vi "LaserPanel.vi"() -> ()   [LabVIEW 2014]
uses:
  <vilib>/event_ctls.llb/eventvkey.ctl
  <vilib>/Instr/_visa.llb/VISA Configure Serial Port (Instr).vi
  wlmData.dll
panel:
  out "Oscilloscope Error":errorcluster
  in  "RF Low":bool=TRUE
  out "Numeric":dbl
  out "Saes Error":errorcluster
  out "Ion\nPump":string="0 nA"
  out "Trap RF error":errorcluster
  out "Horn Error":errorcluster
  out "Cureent error":errorcluster
  out "Oven error":errorcluster
  out "aruduino error":errorcluster
  out "PMT 2":dbl=70.0 format="%.2f"
  in  "DeviceTab":T1(tab)
  in  "Brightness":dbl=30.0
  out "ERROR":string
  in  "Show WLM APP":bool=TRUE
  in  "stop 2":bool
  in  "Expo.[ms]":i32[](array[numeric])
  out "Pattern":i16[][](graph)
  out "Pattern2":i16[][](graph)
  in  "Auto":bool
  in  "Use":bool=TRUE
  in  "stop 3":bool
  out "PID Warning":bool
  out "Act Wavelength (nm)":string
  in  "PID gains":T2={"Pg (Kc)"=1000.0, "It (Ti, min)"=0.0, "Dt (Td, min)"=0.0} {"Dt (Td, min)" format="%.3f"; "It (Ti, min)" format="%.3f"; "Pg (Kc)" format="%.3f"}
  out "Warning":bool
  in  "Set Voltage (V)":dbl=70.0 min=50.0 max=90.0 format="%.3f"
  in  "Set Current  (mA)":dbl=70.0 format="%.3f"
  in  "Set Temperature":dbl=70.0 format="%.3f"
  out "Act Voltage (V)":dbl=70.0 format="%.3f"
  in  "Laser":i16(ring) items=["370", "399", "729", "935"]
  in  "Lock":bool
  in  "Set Wavelength (nm)":dbl=70.0 format="%.6f"
  out "Act Current (mA)":dbl=70.0 format="%.1f"
  out "Max Current (mA)":dbl=70.0 format="%.3f"
  out "Act Temperature":dbl=70.0 format="%.3f"
  in  "RF OFF":bool=TRUE
  in  "Oven+399/SPACE":bool
  in  "Ion refind":bool
  in  "Ion Capture":bool
  out "output 1":dbl
  in  "Ch2 Scale":dbl(ring)=0.5 items=["10V"=10.0, "5V"=5.0, "2V"=2.0, "1V"=1.0, "500mV"=0.5, "200mV"=0.2, "100mV"=0.1, "50mV"=0.05, "20mV"=0.02, "10mV"=0.01, "5mV"=0.005, "2mV"=0.002, "1mV"=0.001]
  out "Numeric 2":dbl
  out "Ch2 pk-pk(V)":dbl format="%.3f"
  out "Ch1 pk-pk(V)":dbl format="%.3f"
  out "ERROR2":string caption="ERROR"
  out "trap default":dbl
  in  "VISA Input":string
  out "VISA Output":string
  in  "Amplitude (dBm)":dbl format="%.1f"
  in  "RFon/off":bool caption="ON"
  in  "Amplitude2(dBm)":dbl format="%.1f"
  in  "Frequency (MHz)":dbl format="%.4f"
  in  "Device":i16(ring) items=["Trap", "Horn/Raman"]
  out "ERROR3":string caption="ERROR"
  in  "Track":i16(ring) items=["Indenpent", "Series", "Parallel"]
  out "Temperature":dbl format="%.2f"
  in  "Channel":i16(ring) items=["Oven", "Current1", "Current2", "Current3", "Current4"]
  in  "Con/off":bool caption="ON"
  out "T":dbl(slide) scale=0.0..100.0
  out "CV":bool
  out "CC":bool
  in  "Set Voltage (V)":dbl=1.5 format="%.3f"
  in  "Set Current (A)":dbl=1.3 format="%.3f"
  out "Act Voltage (V)":dbl format="%.3f"
  out "Act Current (A)":dbl format="%.3f"
  out "PMT":dbl=70.0 format="%.2f"
  in  "CCD/F7":bool=TRUE
  in  "935/F6":bool=TRUE
  in  "399":bool=TRUE
  in  "370/F5":bool=TRUE
  in  "Show2":bool=TRUE
  in  "Show4":bool=TRUE
  in  "Show1":bool=TRUE
  in  "Show3":bool=TRUE
  out "Booleanno":bool
  out "Boolean 2":bool
  out "Boolean":bool
  in  "Warning 3":bool
  in  "Warning 2":bool
  in  "Warning 1":bool
  in  "Warning 0":bool
  out "Set Volt Array 0":dbl[](array[numeric])
  out "935":string
  out "729":string
  out "399":string
  out "370":string
  out "Act Wavelength number (nm)":dbl=70.0 format="%.6f"
  out "Set wave Array":dbl[](array[numeric])
  out "Lock Array":bool[](array[boolean])
  in  "stop":bool
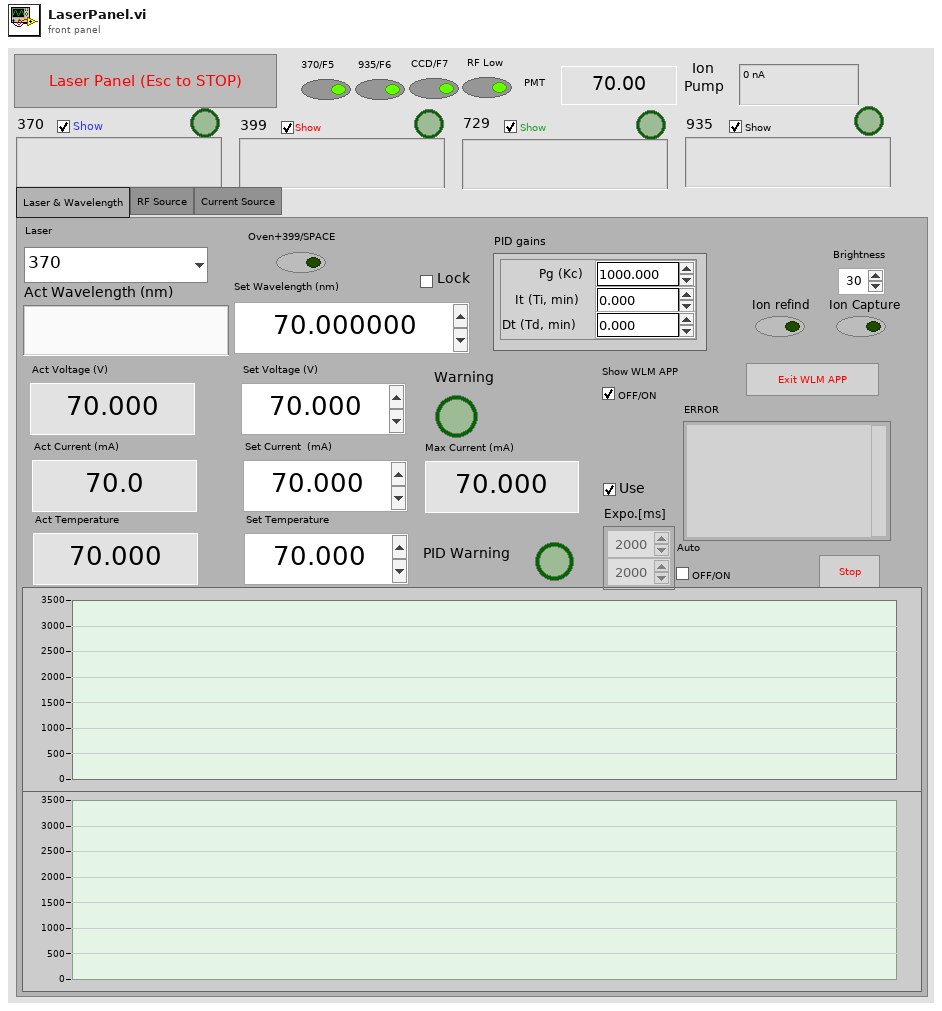
[diagram p1: front panel]
types:
  T1 = enum32{"Laser & Wavelength", "RF Source", "Current Source"}
  T2 = cluster{"Pg (Kc)":dbl, "It (Ti, min)":dbl, "Dt (Td, min)":dbl}
  T3 = typedef "eventvkey.ctl" = enum16{"ASCII", "Enter", "Return", "Shift", "Ctrl", "Alt", "Cmd", "Opt", "Caps", "NumLock", "Clear", "Break", "Up", "Down", "Left", "Right", "Insert", "Delete", "Home", "End", "PageUp", "PageDown", "Escape", "Help", "Pause", "ScrollLock", "F1", "F2", "F3", "F4", "F5", "F6", "F7", "F8", "F9", "F10", "F11", "F12", "F13", "F14", "F15", "F16", "F17", "F18", "F19", "F20", "F21", "F22", "F23", "F24", "Play", "VolumeUp", "VolumeDown", "Mute", "Two Byte Char"}
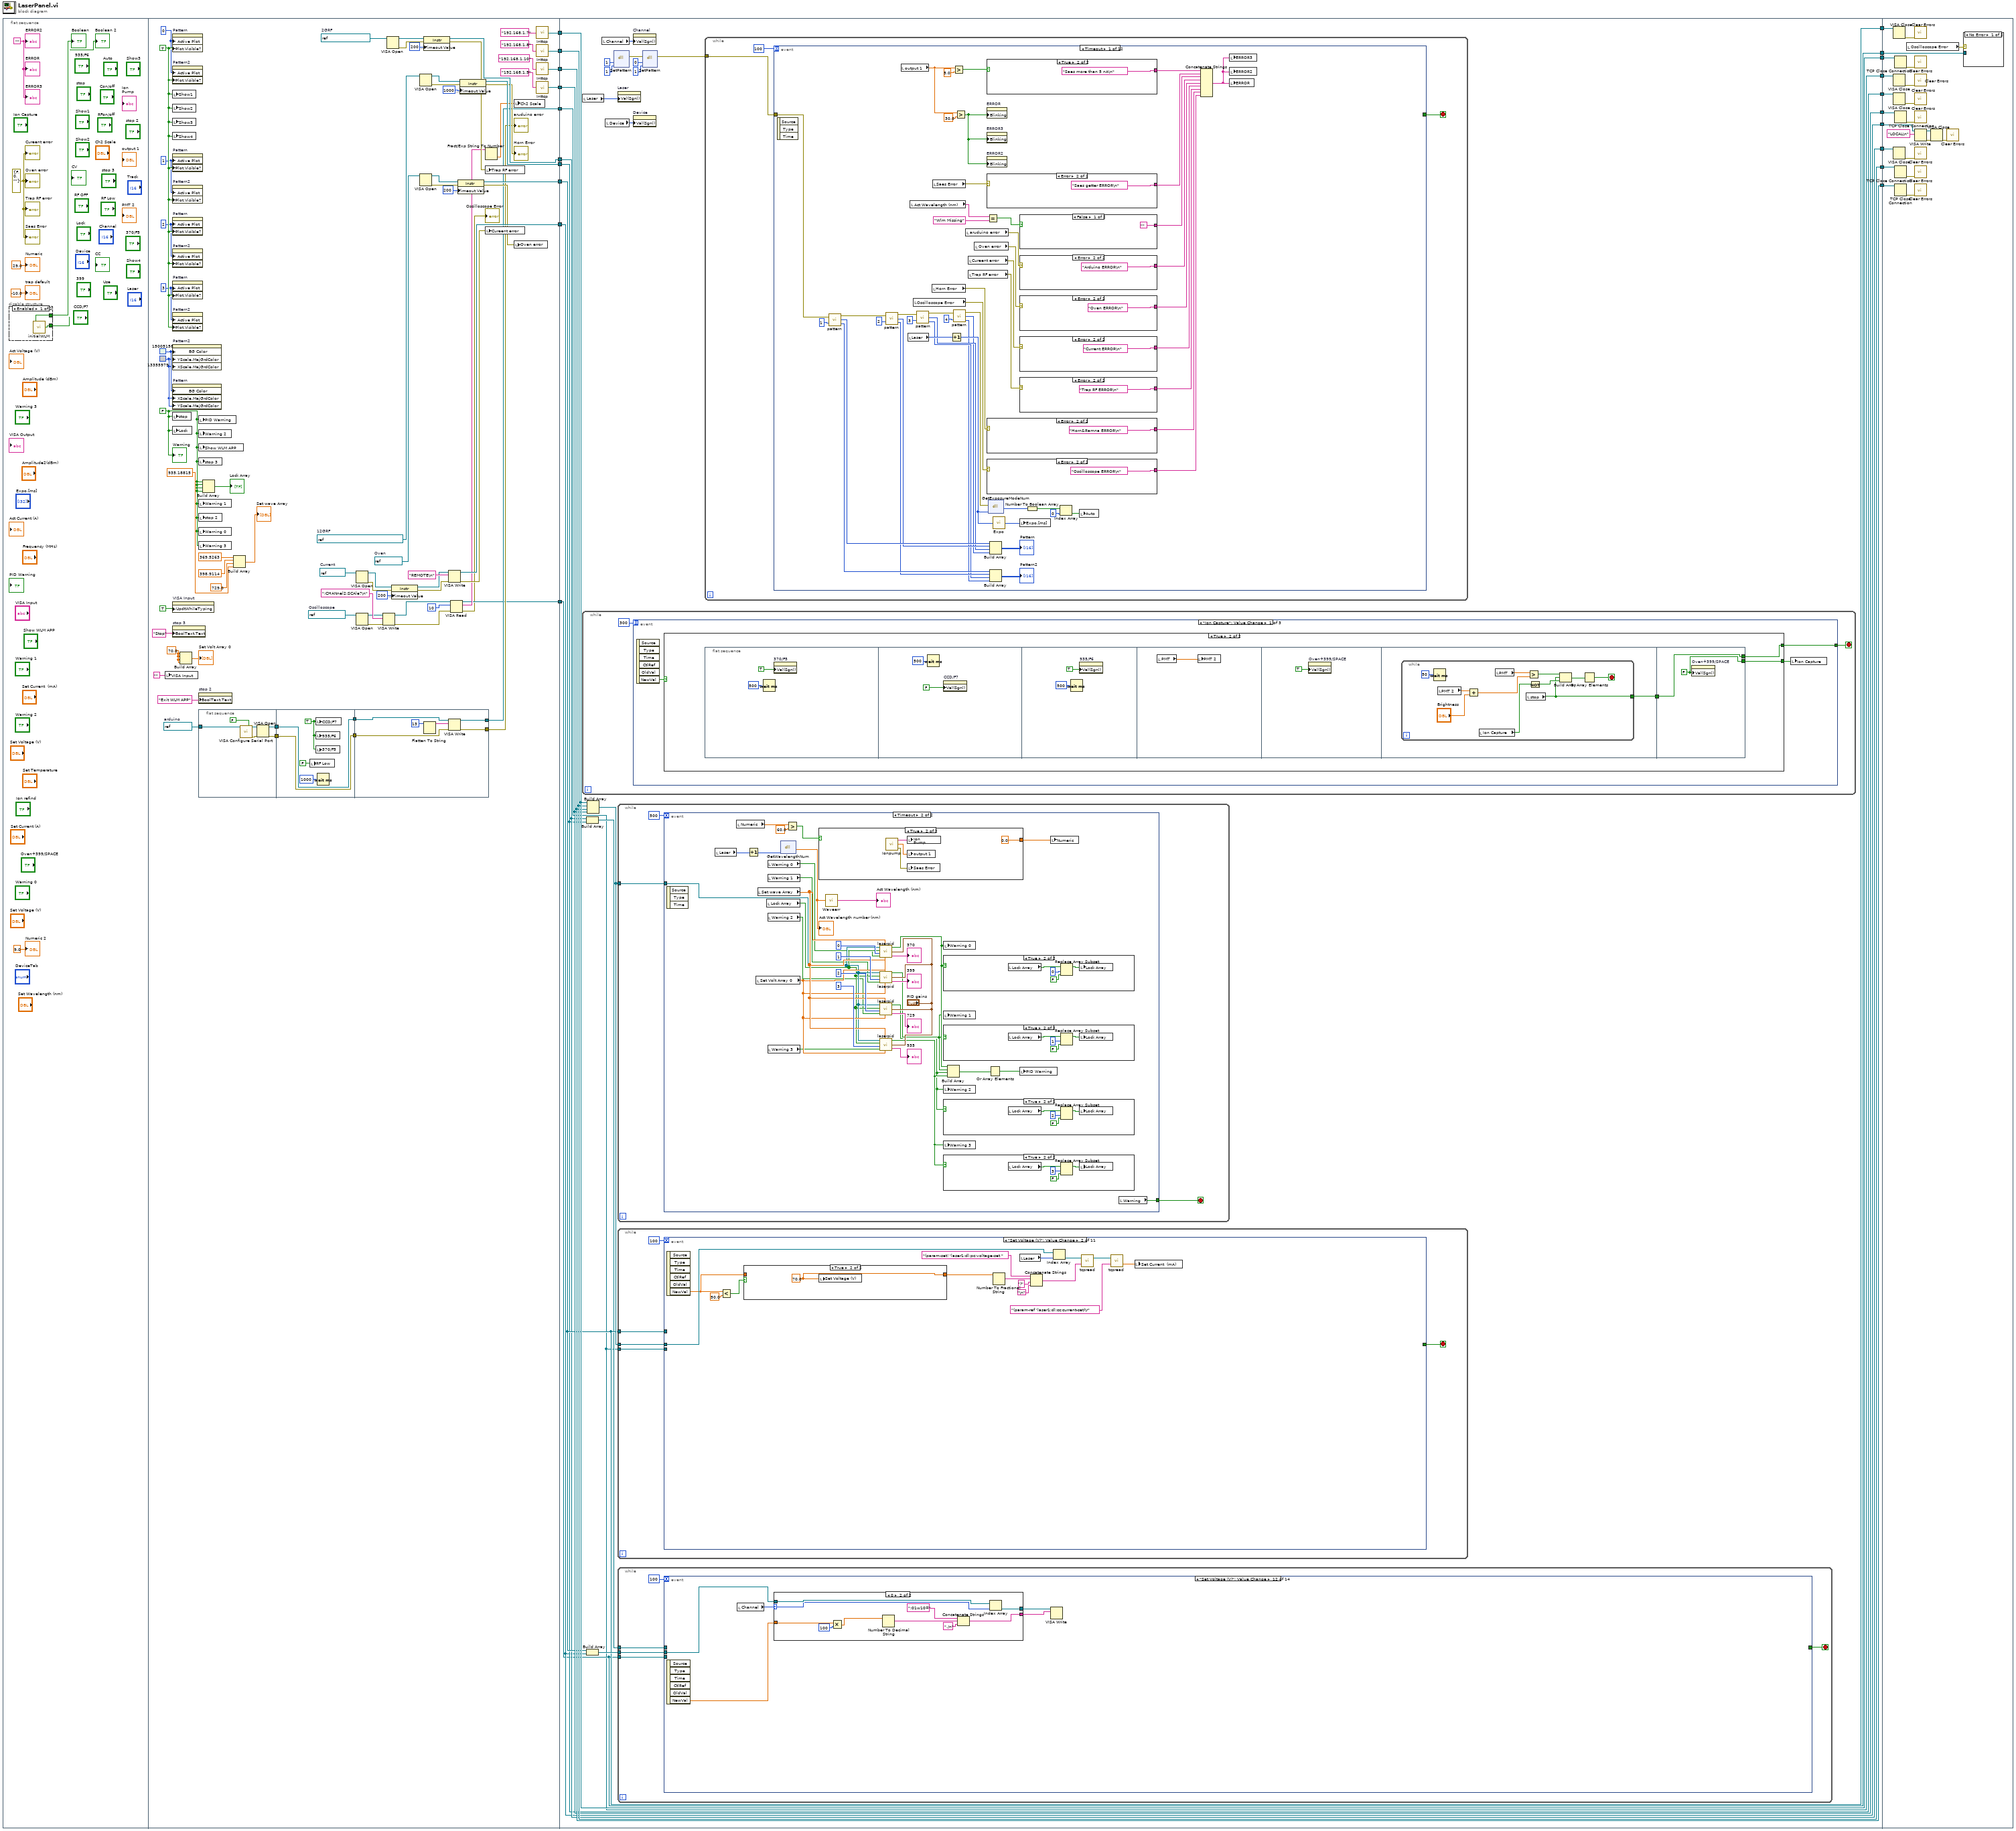
[diagram p0: block diagram]
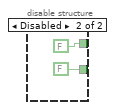
[diagram p2: hidden frame]
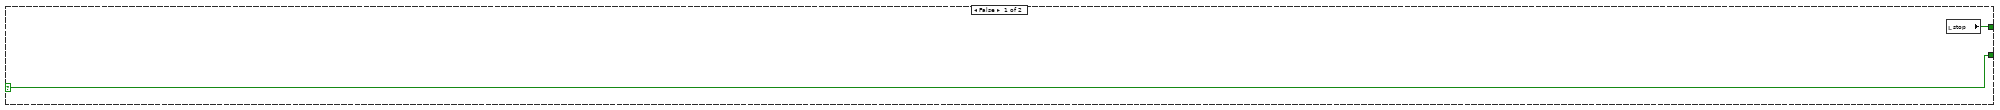
[diagram p3: hidden frame]
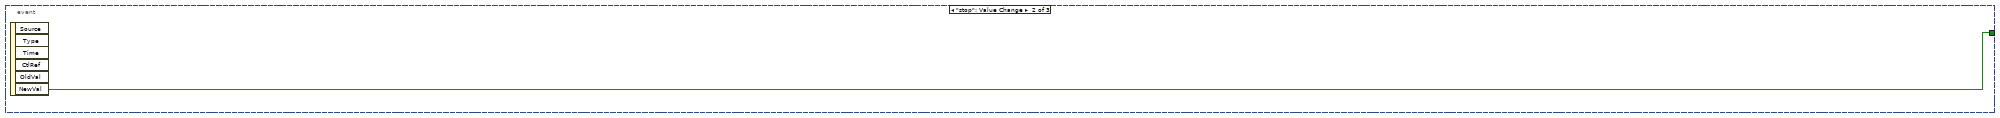
[diagram p4: hidden frame]
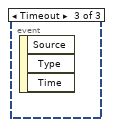
[diagram p5: hidden frame]
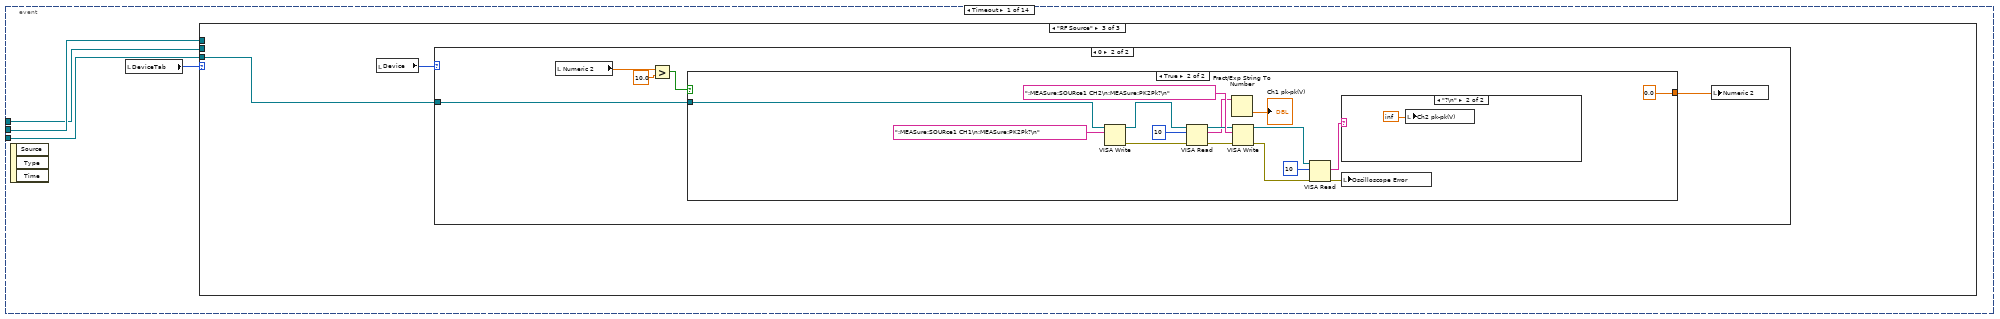
[diagram p6: hidden frame]
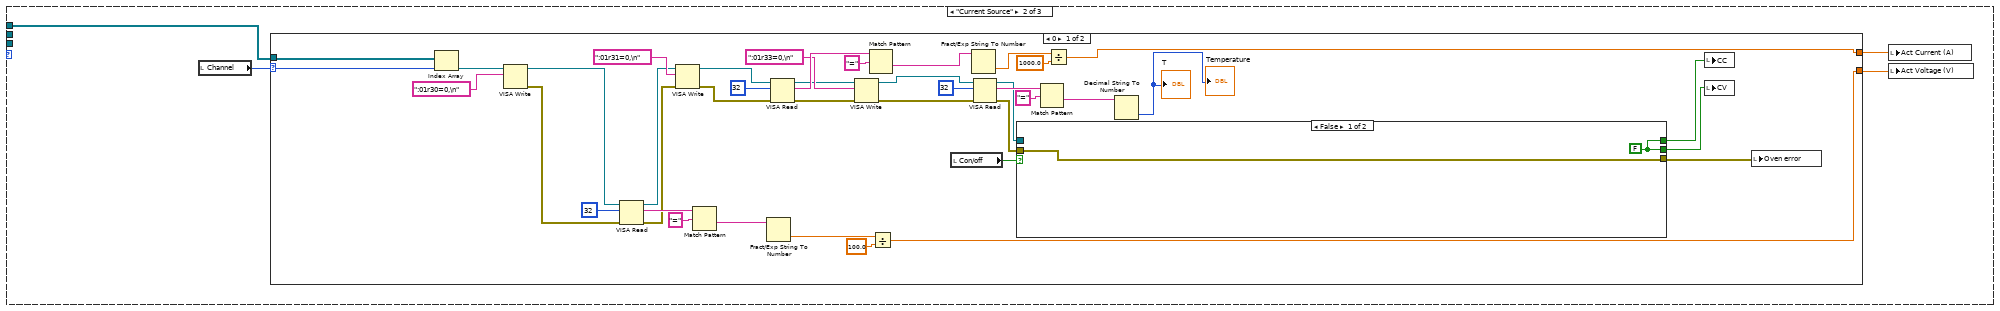
[diagram p8: hidden frame]
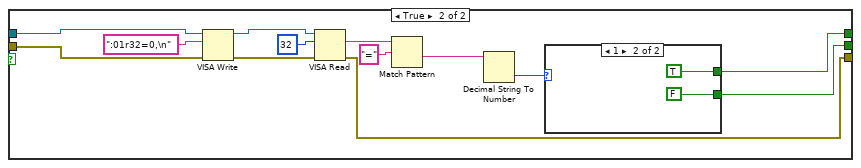
[diagram p9: hidden frame]
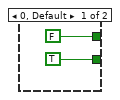
[diagram p10: hidden frame]
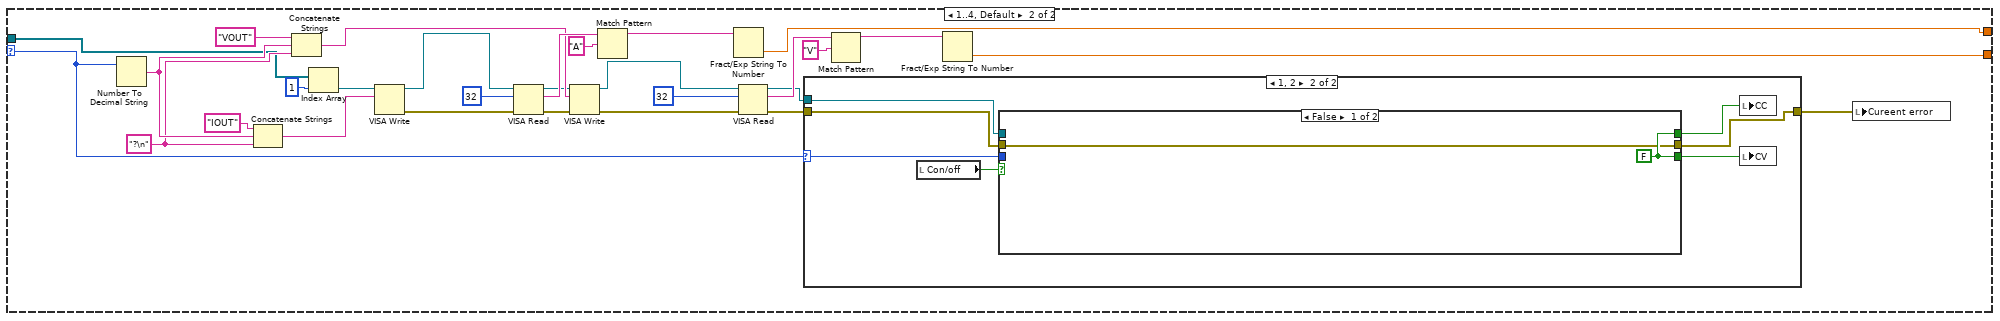
[diagram p11: hidden frame]
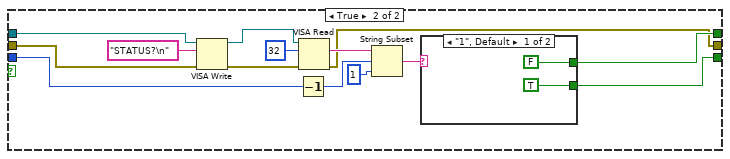
[diagram p13: hidden frame]
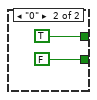
[diagram p14: hidden frame]
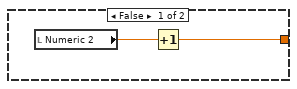
[diagram p16: hidden frame]
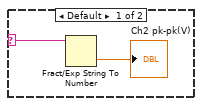
[diagram p17: hidden frame]
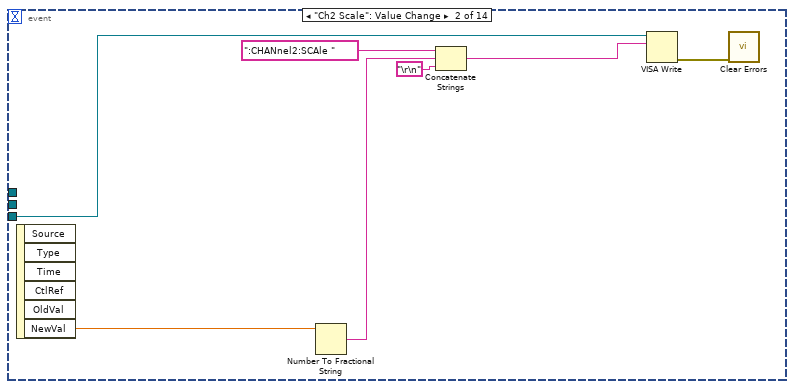
[diagram p18: hidden frame]
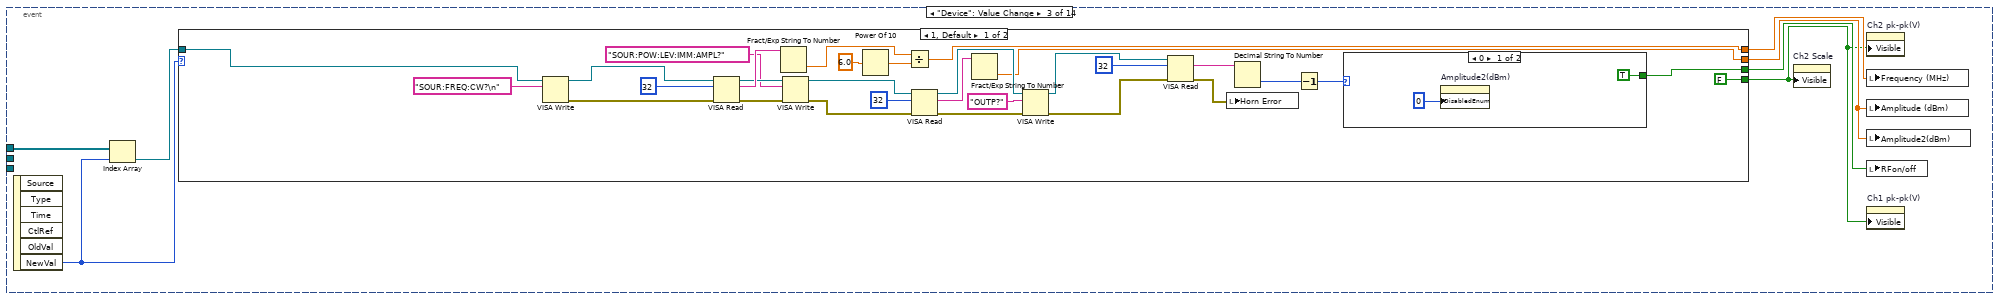
[diagram p19: hidden frame]
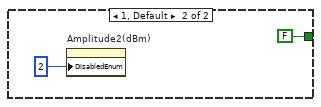
[diagram p20: hidden frame]
diagram:
  n1 = flat-sequence {
    tunnel: [w102] -> w20
    tunnel: [w101] -> w19
    tunnel: [w100] -> w18
    tunnel: [w99] -> w17
    tunnel: [w45] -> w12
    tunnel: [w57] -> w11
    tunnel: [w61] -> w10
    tunnel: [w69] -> w6
    tunnel: [w60] -> w4
    tunnel: [w37] -> w2
    tunnel: w20 -> [w142]
    tunnel: w19 -> [w141]
    tunnel: w18 -> [w140]
    tunnel: w17 -> [w139]
    tunnel: [w142] -> w16
    tunnel: [w141] -> w15
    tunnel: [w140] -> w14
    tunnel: [w139] -> w13
    tunnel: w12 -> [w122]
    tunnel: w11 -> [w130]
    tunnel: w10 -> [w129]
    tunnel: [w122] -> w9
    tunnel: [w130] -> w8
    tunnel: [w129] -> w7
    tunnel: w6 -> [w125]
    tunnel: [w125] -> w5
    tunnel: w4 -> [w124]
    tunnel: [w124] -> w3
    tunnel: w2 -> [w123]
    tunnel: [w123] -> w1
    tunnel: w16 -> [w1110]
    tunnel: w15 -> [w1109]
    tunnel: w14 -> [w1108]
    tunnel: w13 -> [w1107]
    tunnel: w9 -> [w1106]
    tunnel: w8 -> [w1105]
    tunnel: w7 -> [w1104]
    tunnel: w5 -> [w1103]
    tunnel: w3 -> [w1101]
    tunnel: w1 -> [w1099]
    frame #0 {
      w22 = ""
      w24 = errorcluster {"status"=FALSE, "code"=0, "source"=""} ("aruduino error 4")
      n2 = disable-structure shown="Enabled" {
        disable-tunnel: [w29 FALSE] -> w27
        disable-tunnel: [w28 FALSE] -> w26
        frame Enabled {
          n3 = call "initialWLM.vi"() -> ("Boolean 2"=w28:bool, "Boolean"=w29:bool)
        }
        frame Disabled {
        }
      }
      "Boolean" <- w27
      "Boolean 2" <- w26
      "trap default" <- -10.0
      "ERROR" <- w22
      "Trap RF error" <- w24
      "Cureent error" <- w24
      "Oven error" <- w24
      "ERROR2" <- w22
      "ERROR3" <- w22
      "Saes Error" <- w24
      "Numeric" <- 29.0
      "Numeric 2" <- 9.0
    }
    frame #1 {
      w52 = refnum<visa-resource-name> "GDS-1104B"  # Oscilloscope
      w68 = refnum<visa-resource-name> "COM7"  # Current
      w72 = refnum<visa-resource-name> "TCPIP0::192.168.1.11::inst0::INSTR"  # 12GRF
      w77 = refnum<visa-resource-name> "GPIB0::28::INSTR"  # 2GRF
      w78 = refnum<visa-resource-name> "COM16"  # Oven
      w79 = refnum<visa-resource-name> "COM21"  # arduino
      w84 = TRUE
      w81 = 2
      w80 = 3
      w82 = 1
      w83 = 0
      w87 = u32 13355979 ("Color Box")
      w88 = u32 15005158
      w91 = 70.0
      w48 = FALSE
      n4 = local write "VISA Input"("") -> ()
      n5 = property on="Pattern" class="WFGraph (strict)"("Active Plot"=w83, "Plot.Visible?"=w84) -> ()  [unwired: 2 in, 2 out]
      n6 = property on="Pattern2" class="WFGraph (strict)"("Active Plot"=w83, "Plot.Visible?"=w84) -> ()  [unwired: 2 in, 2 out]
      n7 = local write "Show1"(w84) -> ()
      n8 = local write "Show2"(w84) -> ()
      n9 = local write "Show3"(w84) -> ()
      n10 = local write "Show4"(w84) -> ()
      n11 = property on="Pattern" class="WFGraph (strict)"("Active Plot"=w82, "Plot.Visible?"=w84) -> ()  [unwired: 2 in, 2 out]
      n12 = property on="Pattern2" class="WFGraph (strict)"("Active Plot"=w82, "Plot.Visible?"=w84) -> ()  [unwired: 2 in, 2 out]
      n13 = property on="Pattern" class="WFGraph (strict)"("Active Plot"=w81, "Plot.Visible?"=w84) -> ()  [unwired: 2 in, 2 out]
      n14 = property on="Pattern2" class="WFGraph (strict)"("Active Plot"=w81, "Plot.Visible?"=w84) -> ()  [unwired: 2 in, 2 out]
      n15 = property on="Pattern" class="WFGraph (strict)"("Active Plot"=w80, "Plot.Visible?"=w84) -> ()  [unwired: 2 in, 2 out]
      n16 = property on="Pattern2" class="WFGraph (strict)"("Active Plot"=w80, "Plot.Visible?"=w84) -> ()  [unwired: 2 in, 2 out]
      n17 = property on="Pattern2" class="WFGraph (strict)"("BG Color"=w88, "YScale.MajGrdColor"=w87, "XScale.MajGrdColor"=w87) -> ()  [unwired: 2 in, 2 out]
      n18 = property on="Pattern" class="WFGraph (strict)"("BG Color"=w88, "XScale.MajGrdColor"=w87, "YScale.MajGrdColor"=w87) -> ()  [unwired: 2 in, 2 out]
      n19 = local write "stop"(w48) -> ()
      n20 = local write "Lock"(w48) -> ()
      n21 = property on="VISA Input" class="Str"("UpdtWhileTyping"=TRUE) -> ()  [unwired: 2 in, 2 out]
      n22 = property on="stop 3" class="Bool (strict)"("BoolText.Text"="Stop") -> ()  [unwired: 2 in, 2 out]
      n23 = Build Array(w91, w91, w91, w91) -> (→"Set Volt Array 0":dbl[])
      n24 = local write "PID Warning"(w48) -> ()
      n25 = local write "Warning 2"(w48) -> ()
      n26 = local write "Show WLM APP"(w48) -> ()
      n27 = local write "stop 3"(w48) -> ()
      n28 = local write "Warning 1"(w48) -> ()
      n29 = local write "stop 2"(w48) -> ()
      n30 = local write "Warning 0"(w48) -> ()
      n31 = local write "Warning 3"(w48) -> ()
      n32 = property on="stop 2" class="Bool (strict)"("BoolText.Text"="Exit WLM APP") -> ()  [unwired: 2 in, 2 out]
      n33 = flat-sequence {
        tunnel: w79 -> [w110]
        tunnel: [w106] -> w46
        tunnel: [w105] -> w43
        tunnel: [w115] -> w47
        tunnel: w46 -> [w115]
        tunnel: [w111] -> w44
        tunnel: w43 -> [w111]
        tunnel: w47 -> [w119]
        tunnel: [w118] -> w45
        tunnel: w44 -> [w117]
        tunnel: [w116] -> w42
        frame #0 {
          n34 = call-poly "VISA Configure Serial Port"("VISA resource name"=w110, "Enable Termination\nChar (T)"=FALSE ("Enable Termination\nChar (T)")) -> ("VISA resource name out"=w108:refnum<visa-resource-name>, "error out"=w107:errorcluster)  [unwired: 12 in]
          n35 = VISA Open(error in (no error)=w107, VISA resource name=w108) -> (VISA resource name=w106:refnum<visa-resource-name>, error out=w105:errorcluster)  [unwired: 3 in]
        }
        frame #1 {
          w113 = TRUE
          n36 = local write "RF Low"(FALSE) -> ()
          n37 = local write "CCD/F7"(w113) -> ()
          n38 = local write "935/F6"(w113) -> ()
          n39 = local write "370/F5"(w113) -> ()
          n40 = Wait (ms)(milliseconds to wait=u32 1000) -> ()  [unwired: 1 out]
        }
        frame #2 {
          n41 = Flatten To String(anything=u8 13) -> (data string=w120:string)  [unwired: 3 in, 2 out]
          n42 = VISA Write(VISA resource name=w119, write buffer=w120, error in (no error)=w117) -> (VISA resource name out=w118:refnum<visa-resource-name>, error out=w116:errorcluster)  [unwired: 1 out]
        }
      }
      n43 = Build Array(w48, w48, w48, w48) -> (→"Lock Array":bool[])
      n44 = Build Array(369.5263, 398.9114, 729.0, 935.18815) -> (→"Set wave Array":dbl[])
      n45 = VISA Open(VISA resource name=w68) -> (VISA resource name=w66:refnum<visa-resource-name>, error out=w64:errorcluster)  [unwired: 4 in]
      n46 = VISA Open(VISA resource name=w52) -> (VISA resource name=w33:refnum<visa-resource-name>, error out=w32:errorcluster)  [unwired: 4 in]
      n47 = VISA Write(VISA resource name=w33, write buffer=":CHANnel2:SCAle?\n", error in (no error)=w32) -> (VISA resource name out=w34:refnum<visa-resource-name>, error out=w36:errorcluster)  [unwired: 1 out]
      n48 = VISA Open(VISA resource name=w77) -> (VISA resource name=w74:refnum<visa-resource-name>, error out=w54:errorcluster)  [unwired: 4 in]
      n49 = property class="Instr"(reference=w66, error in=w64, "General Settings:Timeout Value"=200) -> (reference out=w63:refnum<visa-resource-name>, error out=w62:errorcluster)
      n50 = VISA Open(VISA resource name=w72) -> (VISA resource name=w70:refnum<visa-resource-name>, error out=w56:errorcluster)  [unwired: 4 in]
      n51 = VISA Open(VISA resource name=w78) -> (VISA resource name=w58:refnum<visa-resource-name>, error out=w51:errorcluster)  [unwired: 4 in]
      n52 = property class="Instr"(reference=w74, error in=w54, "General Settings:Timeout Value"=u32 200) -> (reference out=w61:refnum<visa-resource-name>, error out=w53:errorcluster)
      n53 = VISA Write(VISA resource name=w63, write buffer="REMOTE\n", error in (no error)=w62) -> (VISA resource name out=w60:refnum<visa-resource-name>, error out=w49:errorcluster)  [unwired: 1 out]
      n54 = VISA Read(VISA resource name=w34, byte count=10, error in (no error)=w36) -> (VISA resource name out=w37:refnum<visa-resource-name>, read buffer=w41:string, error out=→"Oscilloscope Error":errorcluster)  [unwired: 1 out]
      n55 = property class="Instr"(reference=w58, error in=w51, "General Settings:Timeout Value"=200) -> (reference out=w57:refnum<visa-resource-name>, error out=w50:errorcluster)
      n56 = property class="Instr"(reference=w70, error in=w56, "General Settings:Timeout Value"=u32 1000) -> (reference out=w69:refnum<visa-resource-name>, error out=→"Horn Error":errorcluster)
      n57 = Fract/Exp String To Number(string=w41) -> (number=w38:dbl)  [unwired: 3 in, 1 out]
      n58 = local write "Trap RF error"(w53) -> ()
      n59 = local write "Cureent error"(w49) -> ()
      n60 = local write "Ch2 Scale"(w38) -> ()
      n61 = local write "Oven error"(w50) -> ()
      n62 = call "Inttcp.vi"("String"="192.168.1.7" ("address")) -> ("TCP Network Connection Refnum"=w102:refnum<k5>)
      n63 = call "Inttcp.vi"("String"="192.168.1.8" ("address")) -> ("TCP Network Connection Refnum"=w101:refnum<k5>)
      n64 = call "Inttcp.vi"("String"="192.168.1.10" ("address")) -> ("TCP Network Connection Refnum"=w100:refnum<k5>)
      n65 = call "Inttcp.vi"("String"="192.168.1.9" ("address")) -> ("TCP Network Connection Refnum"=w99:refnum<k5>)
      "Warning" <- w48
      "aruduino error" <- w42
    }
    frame #2 {
      n66 = local read "Laser"() -> (w143:i16)
      n67 = while {
        stop <- w145 stop-if-true
        n68 = event shown="[0] \"Ion Capture\": Value Change" {
          selector: _ -> [_ _ _]
          dyn-events: _ -> [_ _ _]
          timeout: 300 -> [_ _ _]
          tunnel: [w146 w176 _] -> w145
          event "Ion Capture": Value Change {
            n69 = event-data() -> ("NewVal"=w148:bool)  [unwired: 1 in, 5 out]
            n70 = case shown="True" w148 {
              selector: w148 -> [w150 _]
              tunnel: [w150 w153] -> w147
              tunnel: [w149 w152] -> w146
              frame False {
                n71 = local read "stop"() -> (w149:bool)
              }
              frame True {
                n72 = flat-sequence {
                  tunnel: [w162] -> w151
                  tunnel: [w175] -> w153
                  tunnel: [w174] -> w152
                  tunnel: w151 -> [w174]
                  frame #0 {
                    n73 = Wait (ms)(milliseconds to wait=500) -> ()  [unwired: 1 out]
                    n74 = property on="370/F5" class="Bool (strict)"("Val(Sgnl)"=TRUE) -> ()  [unwired: 2 in, 2 out]
                  }
                  frame #1 {
                    n75 = Wait (ms)(milliseconds to wait=500) -> ()  [unwired: 1 out]
                    n76 = property on="CCD/F7" class="Bool (strict)"("Val(Sgnl)"=FALSE) -> ()  [unwired: 2 in, 2 out]
                  }
                  frame #2 {
                    n77 = Wait (ms)(milliseconds to wait=500) -> ()  [unwired: 1 out]
                    n78 = property on="935/F6" class="Bool (strict)"("Val(Sgnl)"=TRUE) -> ()  [unwired: 2 in, 2 out]
                  }
                  frame #3 {
                    n79 = local read "PMT"() -> (w160:dbl)
                    n80 = local write "PMT 2"(w160) -> ()
                  }
                  frame #4 {
                    n81 = property on="Oven+399/SPACE" class="Bool (strict)"("Val(Sgnl)"=TRUE) -> ()  [unwired: 2 in, 2 out]
                  }
                  frame #5 {
                    n82 = while {
                      tunnel: [w164] -> w162
                      stop <- w166 stop-if-true
                      n83 = Wait (ms)(milliseconds to wait=50) -> ()  [unwired: 1 out]
                      n84 = local read "PMT 2"() -> (w171:dbl)
                      n85 = Add(x=w171, y="Brightness") -> (x+y=w170:dbl)
                      n86 = local read "Ion Capture"() -> (w169:bool)
                      n87 = local read "PMT"() -> (w172:dbl)
                      n88 = local read "stop"() -> (w164:bool)
                      n89 = Greater?(x=w172, y=w170) -> (0:w168:bool)
                      n90 = Not(x=w169) -> (.not. x?=w167:bool)
                      n91 = Build Array(w168, w164, w167) -> (w165:bool[])
                      n92 = Or Array Elements(Boolean array=w165) -> (logical OR=w166:bool)
                    }
                  }
                  frame #6 {
                    w175 = FALSE
                    n93 = property on="Oven+399/SPACE" class="Bool (strict)"("Val(Sgnl)"=w175) -> ()  [unwired: 2 in, 2 out]
                  }
                }
              }
            }
            n94 = local write "Ion Capture"(w147) -> ()
          }
          event "stop": Value Change {
            n95 = event-data() -> ("NewVal"=w176:bool)  [unwired: 1 in, 5 out]
          }
          event Timeout {
            n96 = event-data() -> ()  [unwired: 1 in, 3 out]
          }
        }
      }
      n97 = Build Array(w129, w125) -> (w128:refnum<visa-resource-name>[])
      n98 = Build Array(w130, w124) -> (w131:refnum<visa-resource-name>[])
      n99 = Build Array(w142, w141, w140, w139) -> (w138:refnum<k5>[])
      n100 = local read "Channel"() -> (w126:i16)
      n101 = local read "Device"() -> (w127:i16)
      n102 = dll-call lib="wlmData.dll" fn="SetPattern"("Index"=1, "enable"=1) -> (error out=w133:errorcluster)  [unwired: 6 in, 1 out]
      n103 = property on="Laser" class="Ring (strict)"("Val(Sgnl)"=w143) -> ()  [unwired: 2 in, 2 out]
      n104 = while {
        tunnel: w138 -> [w859]
        stop <- w860 stop-if-true
        n105 = event shown="[1] Timeout" {
          selector: _ -> [_ _]
          dyn-events: _ -> [_ _]
          timeout: 500 -> [_ _]
          tunnel: [w862 w877] -> w860
          tunnel: w859 -> [_ w880]
          event "stop": Value Change {
            n106 = event-data() -> ("NewVal"=w862:bool)  [unwired: 1 in, 5 out]
          }
          event Timeout {
            n107 = event-data() -> ()  [unwired: 1 in, 3 out]
            n108 = local read "Laser"() -> (w891:i16)
            n109 = local read "Numeric"() -> (w866:dbl)
            n110 = Increment(x=w891) -> (x+1=w892:i16)
            n111 = local read "Set Volt Array 0"() -> (w881:dbl[])
            n112 = local read "Set wave Array"() -> (w882:dbl[])
            n113 = local read "Lock Array"() -> (w879:bool[])
            n114 = local read "Warning 0"() -> (w876:bool)
            n115 = local read "Warning 1"() -> (w875:bool)
            n116 = local read "Warning 2"() -> (w874:bool)
            n117 = local read "Warning 3"() -> (w873:bool)
            n118 = dll-call lib="wlmData.dll" fn="GetWavelengthNum"("channel"=w892) -> ("res"=w893:dbl)  [unwired: 4 in, 2 out]
            "Act Wavelength number (nm)" <- w893
            n119 = Greater?(x=w866, y=60.0) -> (0:w864:bool)
            n120 = case shown="True" w864 {
              tunnel: [w895 0.0] -> w863
              frame False {
                n121 = local read "Numeric"() -> (w896:dbl)
                n122 = Increment(x=w896) -> (x+1=w895:dbl)
              }
              frame True {
                n123 = call "Ionpump.vi"() -> ("Saes Error"=w898:errorcluster, "output 1"=w899:dbl, "Ion\nPump"=w900:string)
                n124 = local write "Ion\nPump"(w900) -> ()
                n125 = local write "output 1"(w899) -> ()
                n126 = local write "Saes Error"(w898) -> ()
              }
            }
            n127 = call "Waveerr.vi"("Numeric"=w893) -> ("String"=→"Act Wavelength (nm)":string)
            n128 = call "laserpid.vi"("TCP Array"=w880, "Set wave Array"=w882, "Lock Array"=w879, "Numeric"=0, "Set volt Array 0"=w881, "waring in"=w876, "PID gains"="PID gains") -> ("warning out"=w872:bool, "wavelenth"=→"370":string)
            n129 = call "laserpid.vi"("TCP Array"=w880, "Set wave Array"=w882, "Lock Array"=w879, "Numeric"=1, "Set volt Array 0"=w881, "waring in"=w875, "PID gains"="PID gains") -> ("warning out"=w871:bool, "wavelenth"=→"399":string)
            n130 = call "laserpid.vi"("TCP Array"=w880, "Set wave Array"=w882, "Lock Array"=w879, "Numeric"=2, "Set volt Array 0"=w881, "waring in"=w874, "PID gains"="PID gains") -> ("warning out"=w869:bool, "wavelenth"=→"729":string)
            n131 = call "laserpid.vi"("TCP Array"=w880, "Set wave Array"=w882, "Lock Array"=w879, "Numeric"=3, "Set volt Array 0"=w881, "waring in"=w873, "PID gains"="PID gains") -> ("warning out"=w870:bool, "wavelenth"=→"935":string)
            n132 = local write "Warning 0"(w872) -> ()
            n133 = case shown="True" w872 {
              frame False {
              }
              frame True {
                n134 = local read "Lock Array"() -> (w907:bool[])
                n135 = Replace Array Subset(array=w907, new element=FALSE, index=0) -> (w906:bool[])
                n136 = local write "Lock Array"(w906) -> ()
              }
            }
            n137 = local write "Warning 1"(w871) -> ()
            n138 = case shown="True" w871 {
              frame False {
              }
              frame True {
                n139 = local read "Lock Array"() -> (w915:bool[])
                n140 = Replace Array Subset(array=w915, new element=FALSE, index=1) -> (w914:bool[])
                n141 = local write "Lock Array"(w914) -> ()
              }
            }
            n142 = local write "Warning 2"(w869) -> ()
            n143 = case shown="True" w869 {
              frame False {
              }
              frame True {
                n144 = local read "Lock Array"() -> (w912:bool[])
                n145 = Replace Array Subset(array=w912, new element=FALSE, index=2) -> (w911:bool[])
                n146 = local write "Lock Array"(w911) -> ()
              }
            }
            n147 = local write "Warning 3"(w870) -> ()
            n148 = case shown="True" w870 {
              frame False {
              }
              frame True {
                n149 = local read "Lock Array"() -> (w904:bool[])
                n150 = Replace Array Subset(array=w904, new element=FALSE, index=3) -> (w903:bool[])
                n151 = local write "Lock Array"(w903) -> ()
              }
            }
            n152 = Build Array(w872, w871, w869, w870) -> (w868:bool[])
            n153 = Or Array Elements(Boolean array=w868) -> (logical OR=w867:bool)
            n154 = local write "PID Warning"(w867) -> ()
            n155 = local write "Numeric"(w863) -> ()
            n156 = local read "Warning"() -> (w877:bool)
          }
        }
      }
      n157 = while {
        tunnel: w138 -> [w919]
        tunnel: w122 -> [w918]
        tunnel: w130 -> [w917]
        stop <- w921 stop-if-true
        n158 = event shown="[1] \"Set Voltage (V)\": Value Change" {
          selector: _ -> [_ _ _ _ _ _ _ _ _ _ _]
          dyn-events: _ -> [_ _ _ _ _ _ _ _ _ _ _]
          timeout: 100 -> [_ _ _ _ _ _ _ _ _ _ _]
          tunnel: [w922 _ _ _ _ _ _ _ _ _ _] -> w921
          tunnel: w919 -> [_ w932 w967 _ _ w999 _ _ w1050 w1058 w1083]
          tunnel: w918 -> [_ _ w953 _ _ _ w1036 _ _ _ _]
          tunnel: w917 -> [_ _ _ w978 _ _ _ _ _ _ _]
          event "stop": Value Change {
            n159 = event-data() -> ("NewVal"=w922:bool)  [unwired: 1 in, 5 out]
          }
          event "Set Voltage (V)": Value Change {
            n160 = event-data() -> ("NewVal"=w924:dbl)  [unwired: 1 in, 5 out]
            n161 = Less?(x=w924, y=50.0) -> (x < y?=w925:bool)
            n162 = case shown="True" w925 {
              tunnel: w924 -> [w938 _]
              tunnel: [w938 w939] -> w923
              frame False {
              }
              frame True {
                w939 = 70.0
                n163 = local write "Set Voltage (V)"(w939) -> ()
              }
            }
            n164 = Number To Fractional String(number=w923) -> (F-format string=w936:string)  [unwired: 3 in]
            n165 = local read "Laser"() -> (w933:i16)
            n166 = Concatenate Strings("(param-set! 'laser1:dl:pc:voltage-set " ("string"), w936, ")" ("string"), "\n") -> (w930:string)
            n167 = Index Array(array=w932, index=w933) -> (element=w931:refnum<k5>)
            n168 = call "tcpread.vi"("String 2"=w930, "TCP Network Connection Refnum"=w931) -> ("TCP Network Connection Refnum 2"=w929:refnum<k5>)  [unwired: 1 out]
            n169 = call "tcpread.vi"("String 2"="(param-ref 'laser1:dl:cc:current-set)\r" ("write buffer"), "TCP Network Connection Refnum"=w929) -> ("OUT"=w927:dbl)  [unwired: 1 out]
            n170 = local write "Set Current  (mA)"(w927) -> ()
          }
          event Timeout {
            n171 = event-data() -> ()  [unwired: 1 in, 3 out]
            n172 = property class="Instr"(reference=w953) -> (reference out=w951:refnum<visa-resource-name>, error out=w941:errorcluster, "Bytes at Port"=w952:u32)  [unwired: 1 in]
            n173 = local read "Ion refind"() -> (w942:bool)
            n174 = VISA Read(VISA resource name=w951, byte count=w952, error in (no error)=w941) -> (read buffer=w950:string, error out=w940:errorcluster)  [unwired: 2 out]
            n175 = call <vilib>:"Clear Errors.vi"("error in (no error)"=w940) -> ()  [unwired: 5 in, 2 out]
            n176 = case shown="True" w942 {
              frame False {
              }
              frame True {
                n177 = local read "CCD/F7"() -> (w969:bool)
                n178 = case shown="False" w969 {
                  frame False {
                    n179 = local read "935/F6"() -> (w970:bool)
                    n180 = case shown="True" w970 {
                      frame False {
                      }
                      frame True {
                        n181 = local read "PMT"() -> (w975:dbl)
                        n182 = local read "370/F5"() -> (w973:bool)
                        n183 = Less?(x=w975, y=50.0) -> (x < y?=w971:bool)
                        n184 = Equal?(x=w971, y=w973) -> (x = y?=w972:bool)
                        n185 = case shown="False" w972 {
                          tunnel: w971 -> [w976 _]
                          frame False {
                            n186 = property on="370/F5" class="Bool (strict)"("Val(Sgnl)"=w976) -> ()  [unwired: 2 in, 2 out]
                          }
                          frame True {
                          }
                        }
                      }
                    }
                  }
                  frame True {
                  }
                }
              }
            }
            n187 = Spreadsheet String To Array(delimiter (Tab)="\r", format string="%d", spreadsheet string=w950, array type (2D Dbl)=dbl[] []) -> (array=w945:dbl[])
            n188 = local read "Laser"() -> (w968:i16)
            n189 = Index Array(array=w967, index=w968) -> (element=w957:refnum<k5>)
            n190 = Add Array Elements(numeric array=w945) -> (sum=w946:dbl)
            n191 = Array Size(array=w945) -> (size(s)=w944:i32)
            n192 = Divide(x=w946, y=w944) -> (x/y=→"PMT":dbl)
            n193 = call "tcpread.vi"("String 2"="(param-ref 'laser1:dl:cc:current-clip)\r", "TCP Network Connection Refnum"=w957) -> ("OUT"=w954:dbl, "TCP Network Connection Refnum 2"=w956:refnum<k5>)
            "Max Current (mA)" <- w954
            n194 = call "tcpread.vi"("String 2"="(param-ref 'laser1:dl:cc:current-act)\r" ("write buffer"), "TCP Network Connection Refnum"=w956) -> ("OUT"=w955:dbl, "TCP Network Connection Refnum 2"=w965:refnum<k5>)
            "Act Current (mA)" <- w955
            n195 = Greater?(x=w955, y=w954) -> (0:w958:bool)
            n196 = call "tcpread.vi"("String 2"="(param-ref 'laser1:dl:tc:temp-act)\r" ("write buffer"), "TCP Network Connection Refnum"=w965) -> ("OUT"=→"Act Temperature":dbl, "TCP Network Connection Refnum 2"=w962:refnum<k5>)
            n197 = local write "Warning"(w958) -> ()
            n198 = call "tcpread.vi"("String 2"="(param-ref 'laser1:dl:pc:voltage-act)\r" ("write buffer"), "TCP Network Connection Refnum"=w962) -> ("OUT"=→"Act Voltage (V)":dbl)  [unwired: 1 out]
          }
          event "Oven+399/SPACE": Value Change {
            n199 = event-data() -> ("NewVal"=w979:bool)  [unwired: 1 in, 5 out]
            n200 = case shown="True" w979 {
              tunnel: [":01w12=0,\n" ":01w12=1,\n"] -> w980
              tunnel: [FALSE TRUE] -> w977
              frame False {
              }
              frame True {
              }
            }
            n201 = VISA Write(VISA resource name=w978, write buffer=w980) -> ()  [unwired: 1 in, 3 out]
            n202 = property on="399" class="Bool (strict)"("Val(Sgnl)"=w977) -> ()  [unwired: 2 in, 2 out]
            n203 = local write "Con/off"(w977) -> ()
          }
          event Key Down {
            n204 = event-data() -> ("ScanCode"=w985:i16)  [unwired: 1 in, 9 out]
            n205 = local read "DeviceTab"() -> (w986:T1)
            n206 = case shown="\"RF Source\", Default" w986 {
              tunnel: w985 -> [w987 _]
              frame "Laser & Wavelength" {
                n207 = case shown="65" w987 {
                  frame 0, Default {
                  }
                  frame 57 {
                    n208 = local read "Oven+399/SPACE"() -> (w989:bool)
                    n209 = Not(x=w989) -> (.not. x?=w988:bool)
                    n210 = property on="Oven+399/SPACE" class="Bool (strict)"("Val(Sgnl)"=w988) -> ()  [unwired: 2 in, 2 out]
                  }
                  frame 63 {
                    n211 = local read "370/F5"() -> (w991:bool)
                    n212 = Not(x=w991) -> (.not. x?=w990:bool)
                    n213 = property on="370/F5" class="Bool (strict)"("Val(Sgnl)"=w990) -> ()  [unwired: 2 in, 2 out]
                  }
                  frame 64 {
                    n214 = local read "935/F6"() -> (w993:bool)
                    n215 = Not(x=w993) -> (.not. x?=w992:bool)
                    n216 = property on="935/F6" class="Bool (strict)"("Val(Sgnl)"=w992) -> ()  [unwired: 2 in, 2 out]
                  }
                  frame 65 {
                    n217 = local read "CCD/F7"() -> (w995:bool)
                    n218 = Not(x=w995) -> (.not. x?=w994:bool)
                    n219 = property on="CCD/F7" class="Bool (strict)"("Val(Sgnl)"=w994) -> ()  [unwired: 2 in, 2 out]
                  }
                }
              }
              frame "RF Source", Default {
              }
            }
          }
          event "Lock": Value Change {
            n220 = event-data() -> ("NewVal"=w1001:bool)  [unwired: 1 in, 5 out]
            n221 = local read "Act Wavelength number (nm)"() -> (w1003:dbl)
            n222 = local read "Laser"() -> (w998:i16)
            n223 = case shown="True" w1001 {
              tunnel: w998 -> [_ w1004]
              frame False {
              }
              frame True {
                n224 = flat-sequence {
                  tunnel: w1004 -> [w1006]
                  frame #0 {
                    n225 = case shown="0, Default" w1006 {
                      tunnel: FALSE -> [w1007 w1008 w1009 w1010]
                      frame 0, Default {
                        n226 = local write "Warning 0"(w1007) -> ()
                      }
                      frame 1 {
                        n227 = local write "Warning 1"(w1008) -> ()
                      }
                      frame 2 {
                        n228 = local write "Warning 2"(w1009) -> ()
                      }
                      frame 3 {
                        n229 = local write "Warning 3"(w1010) -> ()
                      }
                    }
                  }
                  frame #1 {
                    n230 = local read "Warning 0"() -> (w1014:bool)
                    n231 = local read "Warning 1"() -> (w1012:bool)
                    n232 = local read "Warning 2"() -> (w1013:bool)
                    n233 = local read "Warning 3"() -> (w1011:bool)
                    n234 = Build Array(w1014, w1012, w1013, w1011) -> (w1015:bool[])
                    n235 = Or Array Elements(Boolean array=w1015) -> (logical OR=w1016:bool)
                    n236 = local write "PID Warning"(w1016) -> ()
                  }
                }
              }
            }
            n237 = Index Array(array=w999, index=w998) -> (element=w997:refnum<k5>)
            n238 = Greater Than 0?(x=w1003) -> (x > 0?=w1002:bool)
            n239 = case shown="True" w1002 {
              tunnel: w1001 -> [_ w1021]
              tunnel: w998 -> [_ w1018]
              frame False {
                n240 = local write "Lock"(FALSE) -> ()
              }
              frame True {
                n241 = flat-sequence {
                  tunnel: w1018 -> [w1022]
                  tunnel: w1021 -> [w1023]
                  tunnel: [w1023] -> w1020
                  tunnel: [w1022] -> w1019
                  tunnel: w1020 -> [w1028]
                  tunnel: w1019 -> [w1027]
                  frame #0 {
                    n242 = local read "Set Volt Array 0"() -> (w1024:dbl[])
                    n243 = local read "Set Voltage (V)"() -> (w1025:dbl)
                    n244 = Replace Array Subset(array=w1024, new element=w1025, index=w1022) -> (w1026:dbl[])
                    n245 = local write "Set Volt Array 0"(w1026) -> ()
                  }
                  frame #1 {
                    n246 = local read "Lock Array"() -> (w1030:bool[])
                    n247 = Replace Array Subset(array=w1030, new element=w1028, index=w1027) -> (w1029:bool[])
                    n248 = local write "Lock Array"(w1029) -> ()
                  }
                }
              }
            }
            n249 = call "tcpread.vi"("String 2"="(param-ref 'laser1:dl:pc:voltage-set)\r" ("write buffer"), "TCP Network Connection Refnum"=w997) -> ("OUT"=w996:dbl)  [unwired: 1 out]
            n250 = local write "Set Voltage (V)"(w996) -> ()
          }
          event "370/F5", "399", "935/F6", "CCD/F7", "RF Low", "RF OFF": Value Change {
            w1032 = FALSE ("element")
            n251 = event-data() -> ()  [unwired: 1 in, 6 out]
            n252 = local write "Numeric 2"(inf) -> ()
            n253 = local read "CCD/F7"() -> (w1035:bool)
            n254 = local read "RF Low"() -> (w1034:bool)
            n255 = local read "370/F5"() -> (w1042:bool)
            n256 = local read "935/F6"() -> (w1040:bool)
            n257 = local read "399"() -> (w1041:bool)
            n258 = Build Array(w1042, w1041, w1040, w1035, w1032, w1034, w1032, w1032) -> (w1039:bool[])
            n259 = Boolean Array To Number(Boolean array=w1039) -> (number=w1038:u32)
            n260 = Flatten To String(anything=w1038) -> (data string=w1037:string)  [unwired: 3 in, 2 out]
            n261 = VISA Write(VISA resource name=w1036, write buffer=w1037) -> (error out=w1033:errorcluster)  [unwired: 1 in, 2 out]
            n262 = call <vilib>:"Clear Errors.vi"("error in (no error)"=w1033) -> ()  [unwired: 5 in, 2 out]
          }
          event "Set Wavelength (nm)": Value Change {
            n263 = event-data() -> ("NewVal"=w1046:dbl)  [unwired: 1 in, 5 out]
            n264 = local read "Set wave Array"() -> (w1043:dbl[])
            n265 = local read "Laser"() -> (w1044:i16)
            n266 = Replace Array Subset(array=w1043, new element=w1046, index=w1044) -> (w1045:dbl[])
            n267 = local write "Set wave Array"(w1045) -> ()
          }
          event "Set Current  (mA)": Value Change {
            n268 = event-data() -> ("NewVal"=w1047:dbl)  [unwired: 1 in, 5 out]
            n269 = Number To Fractional String(number=w1047) -> (F-format string=w1053:string)  [unwired: 3 in]
            n270 = local read "Laser"() -> (w1051:i16)
            n271 = Concatenate Strings("(param-set! 'laser1:dl:cc:current-set " ("string"), w1053, ")" ("string"), "\n") -> (w1048:string)
            n272 = Index Array(array=w1050, index=w1051) -> (element=w1049:refnum<k5>)
            n273 = call "tcpread.vi"("String 2"=w1048, "TCP Network Connection Refnum"=w1049) -> ()  [unwired: 2 out]
          }
          event "Set Temperature": Value Change {
            n274 = event-data() -> ("NewVal"=w1060:dbl)  [unwired: 1 in, 5 out]
            n275 = Number To Fractional String(number=w1060) -> (F-format string=w1063:string)  [unwired: 3 in]
            n276 = local read "Laser"() -> (w1059:i16)
            n277 = Concatenate Strings("(param-set! 'laser1:dl:tc:temp-set " ("string"), w1063, ")" ("string"), "\n") -> (w1056:string)
            n278 = Index Array(array=w1058, index=w1059) -> (element=w1057:refnum<k5>)
            n279 = call "tcpread.vi"("String 2"=w1056, "TCP Network Connection Refnum"=w1057) -> ()  [unwired: 2 out]
          }
          event "Laser": Value Change {
            n280 = event-data() -> ("NewVal"=w1082:i16)  [unwired: 1 in, 5 out]
            n281 = disable-structure shown="Enabled" {
              frame Enabled {
                n282 = local read "Laser"() -> (w1085:i16)
                n283 = Increment(x=w1085) -> (x+1=w1086:i16)
                n284 = dll-call lib="wlmData.dll" fn="GetSwitcherSignalStates"("Siganal"=w1086) -> ("Use"=w1087:bool, "Booleanno"=→"Booleanno":bool)  [unwired: 7 in, 2 out]
                n285 = local write "Use"(w1087) -> ()
              }
              frame Disabled {
              }
            }
            n286 = local read "Set wave Array"() -> (w1066:dbl[])
            n287 = local read "Lock Array"() -> (w1069:bool[])
            n288 = local read "Laser"() -> (w1065:i16)
            n289 = Index Array(array=w1066, index=w1065) -> (element=w1067:dbl)
            n290 = Index Array(array=w1069, index=w1065) -> (element=w1068:bool)
            n291 = local write "Set Wavelength (nm)"(w1067) -> ()
            n292 = local write "Lock"(w1068) -> ()
            n293 = Index Array(array=w1083, index=w1082) -> (element=w1081:refnum<k5>)
            n294 = call "tcpread.vi"("String 2"="(param-ref 'laser1:dl:cc:current-set)\r" ("write buffer"), "TCP Network Connection Refnum"=w1081) -> ("OUT"=w1079:dbl, "TCP Network Connection Refnum 2"=w1078:refnum<k5>)
            n295 = local write "Set Current  (mA)"(w1079) -> ()
            n296 = call "tcpread.vi"("String 2"="(param-ref 'laser1:dl:tc:temp-set)\r" ("write buffer"), "TCP Network Connection Refnum"=w1078) -> ("OUT"=w1076:dbl, "TCP Network Connection Refnum 2"=w1071:refnum<k5>)
            n297 = local write "Set Temperature"(w1076) -> ()
            n298 = call "tcpread.vi"("String 2"="(param-ref 'laser1:dl:cc:current-clip)\r", "TCP Network Connection Refnum"=w1071) -> ("OUT"=w1072:dbl, "TCP Network Connection Refnum 2"=w1070:refnum<k5>)
            n299 = local write "Max Current (mA)"(w1072) -> ()
            n300 = call "tcpread.vi"("String 2"="(param-ref 'laser1:dl:pc:voltage-set)\r" ("write buffer"), "TCP Network Connection Refnum"=w1070) -> ("OUT"=w1074:dbl)  [unwired: 1 out]
            n301 = local write "Set Voltage (V)"(w1074) -> ()
          }
        }
      }
      n302 = while {
        tunnel: w131 -> [w179]
        tunnel: w128 -> [w178]
        tunnel: w123 -> [w177]
        stop <- w181 stop-if-true
        n303 = event shown="[11] \"Set Voltage (V)\": Value Change" {
          selector: _ -> [_ _ _ _ _ _ _ _ _ _ _ _ _ _]
          dyn-events: _ -> [_ _ _ _ _ _ _ _ _ _ _ _ _ _]
          timeout: 100 -> [_ _ _ _ _ _ _ _ _ _ _ _ _ _]
          tunnel: [_ _ _ _ _ _ _ _ _ _ _ _ _ w721] -> w181
          tunnel: w179 -> [w184 _ _ _ _ _ _ _ w536 w647 w650 w676 w702 _]
          tunnel: w178 -> [w183 _ w346 w422 _ w437 w479 w495 _ _ _ _ _ _]
          tunnel: w177 -> [w182 w337 _ _ _ _ _ _ _ _ _ _ _ _]
          event Timeout {
            n304 = event-data() -> ()  [unwired: 1 in, 3 out]
            n305 = local read "DeviceTab"() -> (w185:T1)
            n306 = case shown="\"RF Source\"" w185 {
              tunnel: w184 -> [_ w189 _]
              tunnel: w183 -> [_ _ _]
              tunnel: w182 -> [_ _ w307]
              frame "Laser & Wavelength", Default {
              }
              frame "Current Source" {
                n307 = local read "Channel"() -> (w188:i16)
                n308 = case shown="0" w188 {
                  selector: w188 -> [w201 w255]
                  tunnel: w189 -> [w203 w265]
                  tunnel: [w198 w257] -> w187
                  tunnel: [w197 w256] -> w186
                  frame 0 {
                    n309 = Index Array(array=w203, index=w201) -> (element=w204:refnum<visa-resource-name>)
                    n310 = VISA Write(VISA resource name=w204, write buffer=":01r30=0,\n") -> (VISA resource name out=w229:refnum<visa-resource-name>, error out=w196:errorcluster)  [unwired: 1 in, 1 out]
                    n311 = VISA Read(VISA resource name=w229, byte count=u32 32, error in (no error)=w196) -> (VISA resource name out=w214:refnum<visa-resource-name>, read buffer=w227:string, error out=w195:errorcluster)  [unwired: 1 out]
                    n312 = VISA Write(VISA resource name=w214, write buffer=":01r31=0,\n", error in (no error)=w195) -> (VISA resource name out=w216:refnum<visa-resource-name>, error out=w194:errorcluster)  [unwired: 1 out]
                    n313 = Match Pattern(string=w227, regular expression="=") -> (after substring=w225:string)  [unwired: 1 in, 3 out]
                    n314 = Fract/Exp String To Number(string=w225) -> (number=w224:dbl)  [unwired: 3 in, 1 out]
                    n315 = VISA Read(VISA resource name=w216, byte count=u32 32, error in (no error)=w194) -> (VISA resource name out=w208:refnum<visa-resource-name>, read buffer=w218:string, error out=w191:errorcluster)  [unwired: 1 out]
                    n316 = VISA Write(VISA resource name=w208, write buffer=":01r33=0,\n", error in (no error)=w191) -> (VISA resource name out=w210:refnum<visa-resource-name>, error out=w190:errorcluster)  [unwired: 1 out]
                    n317 = Match Pattern(string=w218, regular expression="=") -> (after substring=w220:string)  [unwired: 1 in, 3 out]
                    n318 = Divide(x=w224, y=100.0) -> (x/y=w197:dbl)
                    n319 = local read "Con/off"() -> (w200:bool)
                    n320 = Fract/Exp String To Number(string=w220) -> (number=w221:dbl)  [unwired: 3 in, 1 out]
                    n321 = VISA Read(VISA resource name=w210, byte count=u32 32, error in (no error)=w190) -> (VISA resource name out=w199:refnum<visa-resource-name>, read buffer=w213:string, error out=w193:errorcluster)  [unwired: 1 out]
                    n322 = case shown="False" w200 {
                      tunnel: w199 -> [_ w241]
                      tunnel: [w232 w237] -> w206
                      tunnel: [w232 w236] -> w205
                      tunnel: w193 -> [w231 w235]
                      tunnel: [w231 w233] -> w192
                      frame False {
                        w232 = FALSE
                      }
                      frame True {
                        n323 = VISA Write(VISA resource name=w241, write buffer=":01r32=0,\n", error in (no error)=w235) -> (VISA resource name out=w243:refnum<visa-resource-name>, error out=w234:errorcluster)  [unwired: 1 out]
                        n324 = VISA Read(VISA resource name=w243, byte count=u32 32, error in (no error)=w234) -> (read buffer=w245:string, error out=w233:errorcluster)  [unwired: 2 out]
                        n325 = Match Pattern(string=w245, regular expression="=") -> (after substring=w239:string)  [unwired: 1 in, 3 out]
                        n326 = Decimal String To Number(string=w239) -> (number=w240:i32)  [unwired: 2 in, 1 out]
                        n327 = case shown="1" w240 {
                          tunnel: [TRUE FALSE] -> w237
                          tunnel: [FALSE TRUE] -> w236
                          frame 0, Default {
                          }
                          frame 1 {
                          }
                        }
                      }
                    }
                    n328 = Match Pattern(string=w213, regular expression="=") -> (after substring=w207:string)  [unwired: 1 in, 3 out]
                    n329 = Divide(x=w221, y=1000.0) -> (x/y=w198:dbl)
                    n330 = Decimal String To Number(string=w207) -> (number=→"Temperature" →"T":i32)  [unwired: 2 in, 1 out]
                    n331 = local write "CC"(w205) -> ()
                    n332 = local write "CV"(w206) -> ()
                    n333 = local write "Oven error"(w192) -> ()
                  }
                  frame 1..4, Default {
                    w269 = "?\n" ("string")
                    n334 = Number To Decimal String(number=w255) -> (decimal integer string=w270:string)  [unwired: 1 in]
                    n335 = Concatenate Strings("IOUT", w270, w269) -> (w268:string)
                    n336 = Concatenate Strings("VOUT", w270, w269) -> (w267:string)
                    n337 = Index Array(array=w265, index=1) -> (element=w264:refnum<visa-resource-name>)
                    n338 = VISA Write(VISA resource name=w264, write buffer=w268) -> (VISA resource name out=w275:refnum<visa-resource-name>, error out=w254:errorcluster)  [unwired: 1 in, 1 out]
                    n339 = VISA Read(VISA resource name=w275, byte count=u32 32, error in (no error)=w254) -> (VISA resource name out=w263:refnum<visa-resource-name>, read buffer=w272:string, error out=w253:errorcluster)  [unwired: 1 out]
                    n340 = VISA Write(VISA resource name=w263, write buffer=w267, error in (no error)=w253) -> (VISA resource name out=w261:refnum<visa-resource-name>, error out=w252:errorcluster)  [unwired: 1 out]
                    n341 = Match Pattern(string=w272, regular expression="A") -> (before substring=w271:string)  [unwired: 1 in, 3 out]
                    n342 = Fract/Exp String To Number(string=w271) -> (number=w257:dbl)  [unwired: 3 in, 1 out]
                    n343 = VISA Read(VISA resource name=w261, byte count=u32 32, error in (no error)=w252) -> (VISA resource name out=w258:refnum<visa-resource-name>, read buffer=w260:string, error out=w251:errorcluster)  [unwired: 1 out]
                    n344 = case shown="1, 2" w255 {
                      selector: w255 -> [_ w285]
                      tunnel: w258 -> [_ w286]
                      tunnel: w251 -> [w279 w281]
                      tunnel: [w279 w280] -> w250
                      frame 3, 4, Default {
                      }
                      frame 1, 2 {
                        n345 = local read "Con/off"() -> (w282:bool)
                        n346 = case shown="False" w282 {
                          tunnel: w286 -> [_ w300]
                          tunnel: w285 -> [_ w295]
                          tunnel: [w288 w293] -> w284
                          tunnel: [w288 w292] -> w283
                          tunnel: w281 -> [w287 w291]
                          tunnel: [w287 w289] -> w280
                          frame False {
                            w288 = FALSE
                          }
                          frame True {
                            n347 = VISA Write(VISA resource name=w300, write buffer="STATUS?\n" ("string"), error in (no error)=w291) -> (VISA resource name out=w301:refnum<visa-resource-name>, error out=w290:errorcluster)  [unwired: 1 out]
                            n348 = Decrement(x=w295) -> (x-1=w294:i16)
                            n349 = VISA Read(VISA resource name=w301, byte count=u32 32, error in (no error)=w290) -> (read buffer=w298:string, error out=w289:errorcluster)  [unwired: 2 out]
                            n350 = String Subset(string=w298, offset (0)=w294, length (rest)=1) -> (substring=w296:string)
                            n351 = case shown="\"1\", Default" w296 {
                              tunnel: [TRUE FALSE] -> w293
                              tunnel: [FALSE TRUE] -> w292
                              frame "1", Default {
                              }
                              frame "0" {
                              }
                            }
                          }
                        }
                        n352 = local write "CC"(w283) -> ()
                        n353 = local write "CV"(w284) -> ()
                      }
                    }
                    n354 = Match Pattern(string=w260, regular expression="V") -> (before substring=w259:string)  [unwired: 1 in, 3 out]
                    n355 = Fract/Exp String To Number(string=w259) -> (number=w256:dbl)  [unwired: 3 in, 1 out]
                    n356 = local write "Cureent error"(w250) -> ()
                  }
                }
                n357 = local write "Act Current (A)"(w187) -> ()
                n358 = local write "Act Voltage (V)"(w186) -> ()
              }
              frame "RF Source" {
                n359 = local read "Device"() -> (w308:i16)
                n360 = case shown="0" w308 {
                  tunnel: w307 -> [_ w313]
                  frame 1, Default {
                  }
                  frame 0 {
                    n361 = local read "Numeric 2"() -> (w312:dbl)
                    n362 = Greater?(x=w312, y=10.0) -> (0:w310:bool)
                    n363 = case shown="True" w310 {
                      tunnel: w313 -> [_ w331]
                      tunnel: [w314 0.0] -> w309
                      frame False {
                        n364 = local read "Numeric 2"() -> (w315:dbl)
                        n365 = Increment(x=w315) -> (x+1=w314:dbl)
                      }
                      frame True {
                        n366 = VISA Write(VISA resource name=w331, write buffer=":MEASure:SOURce1 CH1\n:MEASure:PK2Pk?\n") -> (VISA resource name out=w327:refnum<visa-resource-name>, error out=w321:errorcluster)  [unwired: 1 in, 1 out]
                        n367 = VISA Read(VISA resource name=w327, byte count=u32 10, error in (no error)=w321) -> (VISA resource name out=w325:refnum<visa-resource-name>, read buffer=w323:string, error out=w320:errorcluster)  [unwired: 1 out]
                        n368 = Fract/Exp String To Number(string=w323) -> (number=→"Ch1 pk-pk(V)":dbl)  [unwired: 3 in, 1 out]
                        n369 = VISA Write(VISA resource name=w325, write buffer=":MEASure:SOURce1 CH2\n:MEASure:PK2Pk?\n", error in (no error)=w320) -> (VISA resource name out=w329:refnum<visa-resource-name>, error out=w319:errorcluster)  [unwired: 1 out]
                        n370 = VISA Read(VISA resource name=w329, byte count=u32 10, error in (no error)=w319) -> (read buffer=w317:string, error out=w316:errorcluster)  [unwired: 2 out]
                        n371 = case shown="\"?\\n\"" w317 {
                          selector: w317 -> [w332 _]
                          frame Default {
                            n372 = Fract/Exp String To Number(string=w332) -> (number=→"Ch2 pk-pk(V)":dbl)  [unwired: 3 in, 1 out]
                          }
                          frame "?\n" {
                            n373 = local write "Ch2 pk-pk(V)"(inf) -> ()
                          }
                        }
                        n374 = local write "Oscilloscope Error"(w316) -> ()
                      }
                    }
                    n375 = local write "Numeric 2"(w309) -> ()
                  }
                }
              }
            }
          }
          event "Ch2 Scale": Value Change {
            n376 = event-data() -> ("NewVal"=w341:dbl)  [unwired: 1 in, 5 out]
            n377 = Number To Fractional String(number=w341) -> (F-format string=w339:string)  [unwired: 3 in]
            n378 = Concatenate Strings(":CHANnel2:SCAle ", w339, "\r\n") -> (w336:string)
            n379 = VISA Write(VISA resource name=w337, write buffer=w336) -> (error out=w335:errorcluster)  [unwired: 1 in, 2 out]
            n380 = call <vilib>:"Clear Errors.vi"("error in (no error)"=w335) -> ()  [unwired: 5 in, 2 out]
          }
          event "Device": Value Change {
            n381 = event-data() -> ("NewVal"=w345:i16)  [unwired: 1 in, 5 out]
            n382 = Index Array(array=w346, index=w345) -> (element=w348:refnum<visa-resource-name>)
            n383 = case shown="1, Default" w345 {
              tunnel: w348 -> [w356 w406]
              tunnel: [w371 w401] -> w347
              tunnel: [w359 w389] -> w344
              tunnel: [w357 w388] -> w343
              tunnel: [FALSE TRUE] -> w342
              frame 1, Default {
                n384 = VISA Write(VISA resource name=w356, write buffer="SOUR:FREQ:CW?\n") -> (VISA resource name out=w376:refnum<visa-resource-name>, error out=w355:errorcluster)  [unwired: 1 in, 1 out]
                n385 = VISA Read(VISA resource name=w376, byte count=u32 32, error in (no error)=w355) -> (VISA resource name out=w368:refnum<visa-resource-name>, read buffer=w375:string, error out=w354:errorcluster)  [unwired: 1 out]
                n386 = Fract/Exp String To Number(string=w375) -> (number=w372:dbl)  [unwired: 3 in, 1 out]
                n387 = VISA Write(VISA resource name=w368, write buffer="SOUR:POW:LEV:IMM:AMPL?", error in (no error)=w354) -> (VISA resource name out=w369:refnum<visa-resource-name>, error out=w353:errorcluster)  [unwired: 1 out]
                n388 = Power Of 10(x=6.0) -> (10^x=w374:dbl)
                n389 = Divide(x=w372, y=w374) -> (x/y=w371:dbl)
                n390 = VISA Read(VISA resource name=w369, byte count=u32 32, error in (no error)=w353) -> (VISA resource name out=w363:refnum<visa-resource-name>, read buffer=w358:string, error out=w352:errorcluster)  [unwired: 1 out]
                n391 = Fract/Exp String To Number(string=w358) -> (number=w357:dbl)  [unwired: 3 in, 1 out]
                n392 = VISA Write(VISA resource name=w363, write buffer="OUTP?", error in (no error)=w352) -> (VISA resource name out=w365:refnum<visa-resource-name>, error out=w351:errorcluster)  [unwired: 1 out]
                n393 = VISA Read(VISA resource name=w365, byte count=u32 32, error in (no error)=w351) -> (read buffer=w362:string, error out=w350:errorcluster)  [unwired: 2 out]
                n394 = local write "Horn Error"(w350) -> ()
                n395 = Decimal String To Number(string=w362) -> (number=w361:i32)  [unwired: 2 in, 1 out]
                n396 = Decrement(x=w361) -> (x-1=w360:i32)
                n397 = case shown="0" w360 {
                  tunnel: [TRUE FALSE] -> w359
                  frame 0 {
                    n398 = property on="Amplitude2(dBm)" class="DigNum (strict)"("DisabledEnum"=0) -> ()  [unwired: 2 in, 2 out]
                  }
                  frame 1, Default {
                    n399 = property on="Amplitude2(dBm)" class="DigNum (strict)"("DisabledEnum"=2) -> ()  [unwired: 2 in, 2 out]
                  }
                }
              }
              frame 0 {
                n400 = VISA Write(VISA resource name=w406, write buffer="RF?\n") -> (VISA resource name out=w408:refnum<visa-resource-name>, error out=w387:errorcluster)  [unwired: 1 in, 1 out]
                n401 = VISA Read(VISA resource name=w408, byte count=u32 32, error in (no error)=w387) -> (VISA resource name out=w395:refnum<visa-resource-name>, read buffer=w405:string, error out=w386:errorcluster)  [unwired: 1 out]
                n402 = VISA Write(VISA resource name=w395, write buffer="LEVEL?\n", error in (no error)=w386) -> (VISA resource name out=w397:refnum<visa-resource-name>, error out=w385:errorcluster)  [unwired: 1 out]
                n403 = Match Pattern(string=w405, regular expression=" ") -> (after substring=w403:string)  [unwired: 1 in, 3 out]
                n404 = Fract/Exp String To Number(string=w403) -> (number=w402:dbl)  [unwired: 3 in, 1 out]
                n405 = VISA Read(VISA resource name=w397, byte count=u32 32, error in (no error)=w385) -> (read buffer=w393:string, error out=w384:errorcluster)  [unwired: 2 out]
                n406 = local write "Trap RF error"(w384) -> ()
                n407 = Power Of 10(x=6.0) -> (10^x=w400:dbl)
                n408 = Match Pattern(string=w393, regular expression=" ") -> (after substring=w392:string, offset past match=w391:i32)  [unwired: 1 in, 2 out]
                n409 = Divide(x=w402, y=w400) -> (x/y=w401:dbl)
                n410 = Less Than 0?(x=w391) -> (x < 0?=w390:bool)
                n411 = case shown="True" w390 {
                  tunnel: w392 -> [w413 _]
                  tunnel: [TRUE FALSE] -> w389
                  tunnel: [w410 w414] -> w388
                  frame False {
                    n412 = Fract/Exp String To Number(string=w413) -> (number=w410:dbl)  [unwired: 3 in, 1 out]
                    n413 = property on="Amplitude2(dBm)" class="DigNum (strict)"("DisabledEnum"=0) -> ()  [unwired: 2 in, 2 out]
                  }
                  frame True {
                    n414 = property on="Amplitude2(dBm)" class="DigNum (strict)"("DisabledEnum"=2) -> ()  [unwired: 2 in, 2 out]
                    n415 = local read "trap default"() -> (w414:dbl)
                  }
                }
              }
            }
            n416 = property on="Ch2 Scale" class="Ring (strict)"("Visible"=w342) -> ()  [unwired: 2 in, 2 out]
            n417 = property on="Ch2 pk-pk(V)" class="DigNum (strict)"("Visible"=w342) -> ()  [unwired: 2 in, 2 out]
            n418 = local write "Frequency (MHz)"(w347) -> ()
            n419 = local write "Amplitude (dBm)"(w343) -> ()
            n420 = local write "Amplitude2(dBm)"(w343) -> ()
            n421 = local write "RFon/off"(w344) -> ()
            n422 = property on="Ch1 pk-pk(V)" class="DigNum (strict)"("Visible"=w342) -> ()  [unwired: 2 in, 2 out]
          }
          event "Amplitude2(dBm)": Value Change {
            n423 = event-data() -> ("NewVal"=w421:dbl)  [unwired: 1 in, 5 out]
            n424 = local read "Device"() -> (w420:i16)
            n425 = Number To Fractional String(number=w421) -> (F-format string=w423:string)  [unwired: 3 in]
            n426 = case shown="0" w420 {
              tunnel: w423 -> [w427 w429]
              tunnel: [w424 w428] -> w418
              frame 0 {
                n427 = Concatenate Strings("LEVEL " ("write buffer"), w427, "DBM\n" ("write buffer")) -> (w424:string)
              }
              frame 1, Default {
                n428 = Concatenate Strings("SOUR:POW:LEV:IMM:AMPL " ("write buffer"), w429) -> (w428:string)
              }
            }
            n429 = Index Array(array=w422, index=w420) -> (element=w419:refnum<visa-resource-name>)
            n430 = VISA Write(VISA resource name=w419, write buffer=w418) -> (error out=w417:errorcluster)  [unwired: 1 in, 2 out]
            n431 = call <vilib>:"Clear Errors.vi"("error in (no error)"=w417) -> ()  [unwired: 5 in, 2 out]
          }
          event "Amplitude (dBm)": Value Change {
            n432 = event-data() -> ("NewVal"=w431:dbl)  [unwired: 1 in, 5 out]
            n433 = local read "RFon/off"() -> (w433:bool)
            n434 = local read "Device"() -> (w432:i16)
            n435 = case shown="1, Default" w432 {
              tunnel: w431 -> [w434 _]
              frame 0 {
                n436 = local write "trap default"(w434) -> ()
              }
              frame 1, Default {
              }
            }
            n437 = case shown="True" w433 {
              tunnel: w431 -> [w435 w436]
              frame False {
                n438 = local write "Amplitude2(dBm)"(w435) -> ()
              }
              frame True {
                n439 = property on="Amplitude2(dBm)" class="DigNum (strict)"("Val(Sgnl)"=w436) -> ()  [unwired: 2 in, 2 out]
              }
            }
          }
          event Key Down {
            n440 = event-data() -> ("VKey"=w439:T3)  [unwired: 1 in, 9 out]
            n441 = local read "DeviceTab"() -> (w438:T1)
            n442 = case shown="\"RF Source\"" w438 {
              tunnel: w439 -> [_ w443]
              tunnel: w437 -> [_ w440]
              frame "Laser & Wavelength", Default {
              }
              frame "RF Source" {
                n443 = Equal?(x=w443, y=eventvkey."Return" ("VKey")) -> (x = y?=w441:bool)
                n444 = case shown="True" w441 {
                  tunnel: w440 -> [_ w447]
                  frame False {
                  }
                  frame True {
                    n445 = local read "VISA Input"() -> (w444:string)
                    n446 = case shown="\"clc\"" w444 {
                      selector: w444 -> [_ w450]
                      tunnel: ["" w463] -> w448
                      tunnel: w447 -> [_ w461]
                      tunnel: [_ w455] -> w445
                      frame "clc" {
                      }
                      frame Default {
                        n447 = local read "Device"() -> (w460:i16)
                        n448 = Concatenate Strings(w450, "\r") -> (w452:string)
                        n449 = Index Array(array=w461, index=w460) -> (element=w459:refnum<visa-resource-name>)
                        n450 = VISA Write(VISA resource name=w459, write buffer=w452) -> (VISA resource name out=w458:refnum<visa-resource-name>, error out=w456:errorcluster)  [unwired: 1 in, 1 out]
                        n451 = Concatenate Strings("> " ("string"), w452) -> (w453:string)
                        n452 = local read "VISA Output"() -> (w462:string)
                        n453 = VISA Read(VISA resource name=w458, byte count=u32 32, error in (no error)=w456) -> (read buffer=w454:string, error out=w455:errorcluster)  [unwired: 2 out]
                        n454 = Concatenate Strings(w462, w453, w454) -> (w463:string)
                      }
                    }
                    n455 = flat-sequence {
                      tunnel: w448 -> [w465]
                      tunnel: w445 -> [w469]
                      tunnel: [w468] -> w446
                      frame #0 {
                        n456 = local write "VISA Output"(w465) -> ()
                      }
                      frame #1 {
                        n457 = local write "VISA Input"("") -> ()
                        n458 = property on="VISA Output" class="Str"("Text.Scroll Position"=inf) -> ()  [unwired: 2 in, 2 out]
                      }
                      frame #2 {
                        n459 = case shown="Error" w469 {
                          selector: w469 -> [w470 w471]
                          tunnel: [w470 w471] -> w468
                          frame No Error {
                          }
                          frame Error {
                            n460 = local read "VISA Output"() -> (w474:string)
                            n461 = Concatenate Strings(w474, "No Output\n") -> (w473:string)
                            n462 = local write "VISA Output"(w473) -> ()
                          }
                        }
                      }
                    }
                    n463 = call <vilib>:"Clear Errors.vi"("error in (no error)"=w446) -> ()  [unwired: 5 in, 2 out]
                  }
                }
              }
            }
          }
          event "Frequency (MHz)": Value Change {
            n464 = event-data() -> ("NewVal"=w476:dbl)  [unwired: 1 in, 5 out]
            n465 = local read "Device"() -> (w477:i16)
            n466 = case shown="0" w477 {
              tunnel: [w484 w487] -> w478
              tunnel: w476 -> [w483 w490]
              frame 0 {
                n467 = Number To Fractional String(number=w483) -> (F-format string=w482:string)  [unwired: 3 in]
                n468 = local write "Numeric 2"(inf) -> ()
                n469 = Concatenate Strings("RF " ("write buffer"), w482, "MHZ\n" ("write buffer")) -> (w484:string)
              }
              frame 1, Default {
                n470 = Multiply(x=w490, y=1000000.0) -> (x*y=w488:dbl)
                n471 = Number To Fractional String(number=w488) -> (F-format string=w491:string)  [unwired: 3 in]
                n472 = Concatenate Strings("SOUR:FREQ:CW ", w491) -> (w487:string)
              }
            }
            n473 = Index Array(array=w479, index=w477) -> (element=w480:refnum<visa-resource-name>)
            n474 = VISA Write(VISA resource name=w480, write buffer=w478) -> (error out=w475:errorcluster)  [unwired: 1 in, 2 out]
            n475 = call <vilib>:"Clear Errors.vi"("error in (no error)"=w475) -> ()  [unwired: 5 in, 2 out]
          }
          event "RFon/off": Value Change {
            n476 = event-data() -> ("NewVal"=w496:bool)  [unwired: 1 in, 5 out]
            n477 = local read "Device"() -> (w493:i16)
            n478 = Index Array(array=w495, index=w493) -> (element=w497:refnum<visa-resource-name>)
            n479 = case shown="0" w493 {
              tunnel: w497 -> [w503 w515]
              tunnel: w496 -> [w502 w517]
              tunnel: [w500 w518] -> w494
              frame 0 {
                n480 = case shown="False" w502 {
                  tunnel: ["LEVEL:OFF" w508] -> w501
                  tunnel: [2 0] -> w500
                  frame False {
                  }
                  frame True {
                    n481 = local read "Amplitude2(dBm)"() -> (w507:dbl)
                    n482 = Number To Fractional String(number=w507) -> (F-format string=w506:string)  [unwired: 3 in]
                    n483 = Concatenate Strings("LEVEL " ("write buffer"), w506, "DBM\n" ("write buffer")) -> (w508:string)
                  }
                }
                n484 = local write "Numeric 2"(inf) -> ()
                n485 = VISA Write(VISA resource name=w503, write buffer=w501) -> (error out=w499:errorcluster)  [unwired: 1 in, 2 out]
                n486 = local write "Trap RF error"(w499) -> ()
              }
              frame 1, Default {
                n487 = case shown="True" w517 {
                  tunnel: [2 0] -> w518
                  tunnel: ["OUTP OFF" "OUTP ON"] -> w516
                  tunnel: w515 -> [w520 w529]
                  tunnel: [w520 w528] -> w514
                  tunnel: [errorcluster {"status"=FALSE, "code"=0, "source"=""} ("error out") w523] -> w512
                  frame False {
                  }
                  frame True {
                    n488 = local read "Amplitude (dBm)"() -> (w526:dbl)
                    n489 = Number To Fractional String(number=w526) -> (F-format string=w525:string)  [unwired: 3 in]
                    n490 = Concatenate Strings("SOUR:POW:LEV:IMM:AMPL " ("write buffer"), w525) -> (w524:string)
                    n491 = VISA Write(VISA resource name=w529, write buffer=w524) -> (VISA resource name out=w528:refnum<visa-resource-name>, error out=w523:errorcluster)  [unwired: 1 in, 1 out]
                  }
                }
                n492 = VISA Write(VISA resource name=w514, write buffer=w516, error in (no error)=w512) -> (error out=w513:errorcluster)  [unwired: 2 out]
                n493 = local write "Horn Error"(w513) -> ()
              }
            }
            n494 = property on="Amplitude2(dBm)" class="DigNum (strict)"("DisabledEnum"=w494) -> ()  [unwired: 2 in, 2 out]
          }
          event "Channel": Value Change {
            n495 = event-data() -> ("NewVal"=w535:i16)  [unwired: 1 in, 5 out]
            n496 = case shown="1..4" w535 {
              selector: w535 -> [w555 w596]
              tunnel: w536 -> [w561 w627]
              tunnel: [w540 w599] -> w534
              tunnel: [w552 w598] -> w533
              tunnel: [w551 w597] -> w532
              frame 0, Default {
                w537 = FALSE
                w539 = TRUE
                n497 = local write "CC"(w537) -> ()
                n498 = local write "CV"(w537) -> ()
                n499 = property on="Track" class="Ring (strict)"("Visible"=w537) -> ()  [unwired: 2 in, 2 out]
                n500 = property on="Track" class="Ring (strict)"("Visible"=w537) -> ()  [unwired: 2 in, 2 out]
                n501 = property on="CV" class="Bool (strict)"("Visible"=w539) -> ()  [unwired: 2 in, 2 out]
                n502 = property on="CC" class="Bool (strict)"("Visible"=w539) -> ()  [unwired: 2 in, 2 out]
                n503 = property on="T" class="Slide (strict)"("Visible"=w539) -> ()  [unwired: 2 in, 2 out]
                n504 = Index Array(array=w561, index=w555) -> (element=w544:refnum<visa-resource-name>)
                n505 = property on="Temperature" class="DigNum (strict)"("Visible"=w539) -> ()  [unwired: 2 in, 2 out]
                n506 = VISA Write(VISA resource name=w544, write buffer=":01r12=0,\n") -> (VISA resource name out=w546:refnum<visa-resource-name>, error out=w543:errorcluster)  [unwired: 1 in, 1 out]
                n507 = VISA Read(VISA resource name=w546, byte count=u32 32, error in (no error)=w543) -> (VISA resource name out=w541:refnum<visa-resource-name>, read buffer=w549:string, error out=w542:errorcluster)  [unwired: 1 out]
                n508 = VISA Write(VISA resource name=w541, write buffer=":01r33=0,\n", error in (no error)=w542) -> (VISA resource name out=w582:refnum<visa-resource-name>, error out=w560:errorcluster)  [unwired: 1 out]
                n509 = Match Pattern(string=w549, regular expression="=") -> (after substring=w550:string)  [unwired: 1 in, 3 out]
                n510 = Decimal String To Number(string=w550) -> (number=w545:i32)  [unwired: 2 in, 1 out]
                n511 = VISA Read(VISA resource name=w582, byte count=u32 32, error in (no error)=w560) -> (VISA resource name out=w554:refnum<visa-resource-name>, read buffer=w585:string, error out=w553:errorcluster)  [unwired: 1 out]
                n512 = VISA Write(VISA resource name=w554, write buffer=":01r10=0,\n", error in (no error)=w553) -> (VISA resource name out=w577:refnum<visa-resource-name>, error out=w559:errorcluster)  [unwired: 1 out]
                n513 = Match Pattern(string=w585, regular expression="=") -> (after substring=w580:string)  [unwired: 1 in, 3 out]
                n514 = Decimal String To Number(string=w580) -> (number=w579:i32)  [unwired: 2 in, 1 out]
                n515 = VISA Read(VISA resource name=w577, byte count=u32 32, error in (no error)=w559) -> (VISA resource name out=w562:refnum<visa-resource-name>, read buffer=w571:string, error out=w558:errorcluster)  [unwired: 1 out]
                n516 = local write "T"(w579) -> ()
                n517 = VISA Write(VISA resource name=w562, write buffer=":01r11=0,\n", error in (no error)=w558) -> (VISA resource name out=w564:refnum<visa-resource-name>, error out=w557:errorcluster)  [unwired: 1 out]
                n518 = Match Pattern(string=w571, regular expression="=") -> (after substring=w573:string)  [unwired: 1 in, 3 out]
                n519 = Fract/Exp String To Number(string=w573) -> (number=w574:dbl)  [unwired: 3 in, 1 out]
                n520 = VISA Read(VISA resource name=w564, byte count=u32 32, error in (no error)=w557) -> (read buffer=w570:string, error out=w556:errorcluster)  [unwired: 2 out]
                n521 = call <vilib>:"Clear Errors.vi"("error in (no error)"=w556) -> ()  [unwired: 5 in, 2 out]
                n522 = Divide(x=w574, y=100.0) -> (x/y=w552:dbl)
                n523 = Match Pattern(string=w570, regular expression="=") -> (after substring=w568:string)  [unwired: 1 in, 3 out]
                n524 = Fract/Exp String To Number(string=w568) -> (number=w567:dbl)  [unwired: 3 in, 1 out]
                n525 = case shown="0, Default" w545 {
                  tunnel: [FALSE TRUE] -> w540
                  frame 0, Default {
                  }
                  frame 1 {
                  }
                }
                n526 = Divide(x=w567, y=1000.0) -> (x/y=w551:dbl)
              }
              frame 1..4 {
                w607 = FALSE
                w614 = "?\n" ("string")
                n527 = Number To Decimal String(number=w596) -> (decimal integer string=w608:string)  [unwired: 1 in]
                n528 = property on="T" class="Slide (strict)"("Visible"=w607) -> ()  [unwired: 2 in, 2 out]
                n529 = Concatenate Strings("ISET", w608, w614) -> (w622:string)
                n530 = Concatenate Strings("VSET", w608, w614) -> (w612:string)
                n531 = property on="Temperature" class="DigNum (strict)"("Visible"=w607) -> ()  [unwired: 2 in, 2 out]
                n532 = Index Array(array=w627, index=1) -> (element=w625:refnum<visa-resource-name>)
                n533 = VISA Write(VISA resource name=w625, write buffer=w622) -> (VISA resource name out=w624:refnum<visa-resource-name>, error out=w593:errorcluster)  [unwired: 1 in, 1 out]
                n534 = VISA Read(VISA resource name=w624, byte count=u32 32, error in (no error)=w593) -> (VISA resource name out=w615:refnum<visa-resource-name>, read buffer=w619:string, error out=w592:errorcluster)  [unwired: 1 out]
                n535 = VISA Write(VISA resource name=w615, write buffer=w612, error in (no error)=w592) -> (VISA resource name out=w616:refnum<visa-resource-name>, error out=w591:errorcluster)  [unwired: 1 out]
                n536 = Match Pattern(string=w619, regular expression="A") -> (before substring=w618:string)  [unwired: 1 in, 3 out]
                n537 = Fract/Exp String To Number(string=w618) -> (number=w597:dbl)  [unwired: 3 in, 1 out]
                n538 = VISA Read(VISA resource name=w616, byte count=u32 32, error in (no error)=w591) -> (VISA resource name out=w600:refnum<visa-resource-name>, read buffer=w610:string, error out=w590:errorcluster)  [unwired: 1 out]
                n539 = VISA Write(VISA resource name=w600, write buffer="STATUS?\n" ("string"), error in (no error)=w590) -> (VISA resource name out=w605:refnum<visa-resource-name>, error out=w589:errorcluster)  [unwired: 1 out]
                n540 = Match Pattern(string=w610, regular expression="V") -> (before substring=w609:string)  [unwired: 1 in, 3 out]
                n541 = Fract/Exp String To Number(string=w609) -> (number=w598:dbl)  [unwired: 3 in, 1 out]
                n542 = VISA Read(VISA resource name=w605, byte count=u32 32, error in (no error)=w589) -> (read buffer=w594:string, error out=w588:errorcluster)  [unwired: 2 out]
                n543 = call <vilib>:"Clear Errors.vi"("error in (no error)"=w588) -> ()  [unwired: 5 in, 2 out]
                n544 = case shown="1, 2, Default" w596 {
                  tunnel: [FALSE TRUE] -> w595
                  tunnel: w594 -> [_ w630]
                  frame 3, 4 {
                  }
                  frame 1, 2, Default {
                    w631 = 2
                    n545 = String Subset(string=w630, offset (0)=w631, length (rest)=w631) -> (substring=w632:string)
                    n546 = case shown="\"10\"" w632 {
                      tunnel: [2 0 1] -> w629
                      frame "10" {
                      }
                      frame "01", Default {
                      }
                      frame "11" {
                      }
                    }
                    n547 = local write "Track"(w629) -> ()
                  }
                }
                n548 = String Subset(string=w594, offset (0)=5, length (rest)=1) -> (substring=w601:string)
                n549 = case shown="\"0\"" w601 {
                  tunnel: [TRUE FALSE] -> w599
                  frame "1", Default {
                  }
                  frame "0" {
                  }
                }
                n550 = property on="CV" class="Bool (strict)"("Visible"=w595) -> ()  [unwired: 2 in, 2 out]
                n551 = property on="CC" class="Bool (strict)"("Visible"=w595) -> ()  [unwired: 2 in, 2 out]
                n552 = property on="Track" class="Ring (strict)"("Visible"=w595) -> ()  [unwired: 2 in, 2 out]
                n553 = property on="Track" class="Ring (strict)"("Visible"=w595) -> ()  [unwired: 2 in, 2 out]
              }
            }
            n554 = local write "Set Voltage (V)"(w533) -> ()
            n555 = local write "Con/off"(w534) -> ()
            n556 = local write "Set Current (A)"(w532) -> ()
          }
          event "Track": Value Change {
            n557 = event-data() -> ("NewVal"=w644:i16)  [unwired: 1 in, 5 out]
            n558 = Number To Decimal String(number=w644) -> (decimal integer string=w643:string)  [unwired: 1 in]
            n559 = local write "Con/off"(FALSE) -> ()
            n560 = Concatenate Strings("TRACK", w643, "\r") -> (w640:string)
            n561 = Index Array(array=w647, index=1) -> (element=w641:refnum<visa-resource-name>)
            n562 = VISA Write(VISA resource name=w641, write buffer=w640) -> ()  [unwired: 1 in, 3 out]
          }
          event "Set Current (A)": Value Change {
            n563 = event-data() -> ("NewVal"=w652:dbl)  [unwired: 1 in, 5 out]
            n564 = local read "Channel"() -> (w648:i16)
            n565 = case shown="1..4" w648 {
              selector: w648 -> [w653 w666]
              tunnel: w652 -> [w660 w669]
              tunnel: [w656 w663] -> w651
              tunnel: w650 -> [w655 w672]
              tunnel: [w654 w671] -> w649
              frame 0, Default {
                n566 = Multiply(x=w660, y=1000) -> (x*y=w658:dbl)
                n567 = Number To Decimal String(number=w658) -> (decimal integer string=w657:string)  [unwired: 1 in]
                n568 = Concatenate Strings(":01w11=", w657, ",/n") -> (w656:string)
                n569 = Index Array(array=w655, index=w653) -> (element=w654:refnum<visa-resource-name>)
              }
              frame 1..4 {
                n570 = Number To Decimal String(number=w666) -> (decimal integer string=w665:string)  [unwired: 1 in]
                n571 = Number To Fractional String(number=w669) -> (F-format string=w668:string)  [unwired: 3 in]
                n572 = Concatenate Strings("ISET", w665, ":" ("string"), w668, "\r") -> (w663:string)
                n573 = Index Array(array=w672, index=1) -> (element=w671:refnum<visa-resource-name>)
              }
            }
            n574 = VISA Write(VISA resource name=w649, write buffer=w651) -> ()  [unwired: 1 in, 3 out]
          }
          event "Set Voltage (V)": Value Change {
            n575 = event-data() -> ("NewVal"=w677:dbl)  [unwired: 1 in, 5 out]
            n576 = local read "Channel"() -> (w674:i16)
            n577 = case shown="0" w674 {
              selector: w674 -> [w683 w690]
              tunnel: [w679 w695] -> w678
              tunnel: w677 -> [w682 w693]
              tunnel: w676 -> [w681 w692]
              tunnel: [w680 w691] -> w675
              frame 1..4, Default {
                n578 = Number To Decimal String(number=w683) -> (decimal integer string=w685:string)  [unwired: 1 in]
                n579 = Number To Fractional String(number=w682) -> (F-format string=w687:string)  [unwired: 3 in]
                n580 = Concatenate Strings("VSET", w685, ":" ("string"), w687, "\r") -> (w679:string)
                n581 = Index Array(array=w681, index=1) -> (element=w680:refnum<visa-resource-name>)
              }
              frame 0 {
                n582 = Multiply(x=w693, y=100) -> (x*y=w697:dbl)
                n583 = Number To Decimal String(number=w697) -> (decimal integer string=w696:string)  [unwired: 1 in]
                n584 = Concatenate Strings(":01w10=", w696, ",/n") -> (w695:string)
                n585 = Index Array(array=w692, index=w690) -> (element=w691:refnum<visa-resource-name>)
              }
            }
            n586 = VISA Write(VISA resource name=w675, write buffer=w678) -> ()  [unwired: 1 in, 3 out]
          }
          event "Con/off": Value Change {
            n587 = event-data() -> ("NewVal"=w704:bool)  [unwired: 1 in, 5 out]
            n588 = local read "Channel"() -> (w700:i16)
            n589 = case shown="0" w700 {
              selector: w700 -> [_ w714]
              tunnel: w704 -> [w708 w718]
              tunnel: [w705 w717] -> w703
              tunnel: w702 -> [w711 w716]
              tunnel: [w709 w715] -> w701
              frame 1..4, Default {
                n590 = case shown="True" w708 {
                  tunnel: ["0\n" "1\n"] -> w706
                  frame False {
                  }
                  frame True {
                  }
                }
                n591 = Concatenate Strings("OUT", w706) -> (w705:string)
                n592 = Index Array(array=w711, index=1) -> (element=w709:refnum<visa-resource-name>)
              }
              frame 0 {
                n593 = case shown="False" w718 {
                  tunnel: [":01w12=0,\n" ":01w12=1,\n"] -> w717
                  frame False {
                  }
                  frame True {
                  }
                }
                n594 = Index Array(array=w716, index=w714) -> (element=w715:refnum<visa-resource-name>)
              }
            }
            n595 = VISA Write(VISA resource name=w701, write buffer=w703) -> ()  [unwired: 1 in, 3 out]
          }
          event "stop": Value Change {
            n596 = event-data() -> ("NewVal"=w721:bool)  [unwired: 1 in, 5 out]
          }
        }
      }
      n597 = property on="Channel" class="Ring (strict)"("Val(Sgnl)"=w126) -> ()  [unwired: 2 in, 2 out]
      n598 = property on="Device" class="Ring (strict)"("Val(Sgnl)"=w127) -> ()  [unwired: 2 in, 2 out]
      n599 = dll-call lib="wlmData.dll" fn="SetPattern"(error in=w133, "Index"=0, "enable"=1) -> (error out=w132:errorcluster)  [unwired: 5 in, 1 out]
      n600 = while {
        tunnel: w132 -> [w722]
        stop <- w724 stop-if-true
        n601 = event shown="[0] Timeout" {
          selector: _ -> [_ _ _ _ _ _ _ _ _ _ _ _]
          dyn-events: _ -> [_ _ _ _ _ _ _ _ _ _ _ _]
          timeout: 100 -> [_ _ _ _ _ _ _ _ _ _ _ _]
          tunnel: [_ _ _ _ _ _ _ _ _ _ _ w832] -> w724
          tunnel: w722 -> [w751 _ _ _ _ _ _ _ _ _ _ _]
          event Timeout {
            n602 = event-data() -> ()  [unwired: 1 in, 3 out]
            n603 = call "pattern.vi"("Error In"=w751, "Numeric"=1) -> ("Error Out"=w756:errorcluster, "Pattern"=w767:i16[], "Pattern 2"=w766:i16[])
            n604 = call "pattern.vi"("Error In"=w756, "Numeric"=2) -> ("Error Out"=w755:errorcluster, "Pattern"=w764:i16[], "Pattern 2"=w763:i16[])
            n605 = local read "output 1"() -> (w728:dbl)
            n606 = local read "Laser"() -> (w770:i16)
            n607 = local read "Act Wavelength (nm)"() -> (w749:string)
            n608 = local read "Oscilloscope Error"() -> (w726:errorcluster)
            n609 = call "pattern.vi"("Error In"=w755, "Numeric"=3) -> ("Error Out"=w754:errorcluster, "Pattern"=w760:i16[], "Pattern 2"=w758:i16[])
            n610 = local read "Horn Error"() -> (w737:errorcluster)
            n611 = local read "Saes Error"() -> (w727:errorcluster)
            n612 = Increment(x=w770) -> (x+1=w769:i16)
            n613 = Greater?(x=w728, y=5.0) -> (0:w733:bool)
            n614 = call "pattern.vi"("Error In"=w754, "Numeric"=4) -> ("Error Out"=w750:errorcluster, "Pattern"=w759:i16[], "Pattern 2"=w757:i16[])
            n615 = Greater?(x=w728, y=30.0) -> (0:w729:bool)
            n616 = local read "aruduino error"() -> (w746:errorcluster)
            n617 = local read "Cureent error"() -> (w741:errorcluster)
            n618 = local read "Trap RF error"() -> (w739:errorcluster)
            n619 = local read "Oven error"() -> (w743:errorcluster)
            n620 = case shown="True" w733 {
              tunnel: ["" "Saes more than 5 nA\n"] -> w731
              frame False {
              }
              frame True {
              }
            }
            n621 = property on="ERROR" class="Str"("Blinking"=w729) -> ()  [unwired: 2 in, 2 out]
            n622 = property on="ERROR3" class="Str"("Blinking"=w729) -> ()  [unwired: 2 in, 2 out]
            n623 = property on="ERROR2" class="Str"("Blinking"=w729) -> ()  [unwired: 2 in, 2 out]
            n624 = case shown="Error" w727 {
              tunnel: ["" "Saes getter ERROR\n"] -> w734
              frame No Error {
              }
              frame Error {
              }
            }
            n625 = case shown="Error" w737 {
              tunnel: ["" "Horn&Ramna ERROR\n"] -> w736
              frame No Error {
              }
              frame Error {
              }
            }
            n626 = case shown="Error" w726 {
              tunnel: ["" "Oscilloscope ERROR\n"] -> w725
              frame No Error {
              }
              frame Error {
              }
            }
            n627 = Equal?(x=w749, y="Wlm Missing" ("String")) -> (x = y?=w747:bool)
            n628 = dll-call lib="wlmData.dll" fn="GetExposureModeNum"(error in=w750, "num"=w769) -> ("res"=w775:i32)  [unwired: 3 in, 2 out]
            n629 = Build Array(w767, w764, w760, w759) -> (→"Pattern":i16[][])
            n630 = Build Array(w766, w763, w758, w757) -> (→"Pattern2":i16[][])
            n631 = call "Expo.vi"("Numeric"=w769) -> ("Array"=w771:i32[])
            n632 = case shown="False" w747 {
              tunnel: ["" "WLM ERROR\n"] -> w745
              frame False {
              }
              frame True {
              }
            }
            n633 = case shown="Error" w746 {
              tunnel: ["" "Arduino ERROR\n"] -> w744
              frame No Error {
              }
              frame Error {
              }
            }
            n634 = case shown="Error" w743 {
              tunnel: ["" "Oven ERROR\n"] -> w742
              frame No Error {
              }
              frame Error {
              }
            }
            n635 = case shown="Error" w741 {
              tunnel: ["" "Current ERROR\n"] -> w740
              frame No Error {
              }
              frame Error {
              }
            }
            n636 = case shown="Error" w739 {
              tunnel: ["" "Trap RF ERROR\n"] -> w738
              frame No Error {
              }
              frame Error {
              }
            }
            n637 = local write "Expo.[ms]"(w771) -> ()
            n638 = Number To Boolean Array(number=w775) -> (Boolean array=w774:bool[])
            n639 = Index Array(array=w774, index=0) -> (element=w773:bool)
            n640 = local write "Auto"(w773) -> ()
            n641 = Concatenate Strings(w731, w734, w745, w744, w742, w740, w738, w736, w725) -> (w735:string)
            n642 = local write "ERROR3"(w735) -> ()
            n643 = local write "ERROR2"(w735) -> ()
            n644 = local write "ERROR"(w735) -> ()
          }
          event "Show1": Value Change {
            w795 = 0
            n645 = event-data() -> ("NewVal"=w794:bool)  [unwired: 1 in, 5 out]
            n646 = property on="Pattern" class="WFGraph (strict)"("Active Plot"=w795, "Plot.Visible?"=w794) -> ()  [unwired: 2 in, 2 out]
            n647 = property on="Pattern2" class="WFGraph (strict)"("Active Plot"=w795, "Plot.Visible?"=w794) -> ()  [unwired: 2 in, 2 out]
          }
          event "Show2": Value Change {
            w796 = 1
            n648 = event-data() -> ("NewVal"=w797:bool)  [unwired: 1 in, 5 out]
            n649 = property on="Pattern" class="WFGraph (strict)"("Active Plot"=w796, "Plot.Visible?"=w797) -> ()  [unwired: 2 in, 2 out]
            n650 = property on="Pattern2" class="WFGraph (strict)"("Active Plot"=w796, "Plot.Visible?"=w797) -> ()  [unwired: 2 in, 2 out]
          }
          event "Show3": Value Change {
            w798 = 2
            n651 = event-data() -> ("NewVal"=w799:bool)  [unwired: 1 in, 5 out]
            n652 = property on="Pattern" class="WFGraph (strict)"("Active Plot"=w798, "Plot.Visible?"=w799) -> ()  [unwired: 2 in, 2 out]
            n653 = property on="Pattern2" class="WFGraph (strict)"("Active Plot"=w798, "Plot.Visible?"=w799) -> ()  [unwired: 2 in, 2 out]
          }
          event "Show4": Value Change {
            w800 = 3
            n654 = event-data() -> ("NewVal"=w801:bool)  [unwired: 1 in, 5 out]
            n655 = property on="Pattern" class="WFGraph (strict)"("Active Plot"=w800, "Plot.Visible?"=w801) -> ()  [unwired: 2 in, 2 out]
            n656 = property on="Pattern2" class="WFGraph (strict)"("Active Plot"=w800, "Plot.Visible?"=w801) -> ()  [unwired: 2 in, 2 out]
          }
          event "stop 2": Value Change {
            n657 = event-data() -> ("NewVal"=w803:bool)  [unwired: 1 in, 5 out]
            n658 = case shown="True" w803 {
              tunnel: ["Exit WLM APP" "Start WLM APP"] -> w802
              frame False {
                n659 = call "initialWLM.vi"() -> ()  [unwired: 2 out]
              }
              frame True {
                n660 = dll-call lib="wlmData.dll" fn="ControlWLM"("action"=3, "app"=0, "ver"=0) -> ()  [unwired: 7 in, 2 out]
              }
            }
            n661 = property on="stop 2" class="Bool (strict)"("BoolText.Text"=w802) -> ()  [unwired: 2 in, 2 out]
          }
          event "stop 3": Value Change {
            w811 = u16 1 items=["GetText", "Click"] ("Message")
            n662 = event-data() -> ("NewVal"=w810:bool)  [unwired: 1 in, 5 out]
            n663 = case shown="False" w810 {
              tunnel: ["Stop" "Start"] -> w809
              frame False {
              }
              frame True {
              }
            }
            n664 = call "FindButton.vi"() -> ("Handle"=w812:u64)
            n665 = call "startstop.vi"("Message"=w811, "Handle"=w812) -> ()  [unwired: 1 in, 1 out]
            n666 = property on="stop 3" class="Bool (strict)"("BoolText.Text"=w809) -> ()  [unwired: 2 in, 2 out]
          }
          event "Show WLM APP": Value Change {
            n667 = event-data() -> ("NewVal"=w816:bool)  [unwired: 1 in, 5 out]
            n668 = case shown="True" w816 {
              tunnel: [2 1] -> w815
              frame False {
              }
              frame True {
              }
            }
            n669 = dll-call lib="wlmData.dll" fn="ControlWLM"("action"=w815, "app"=0, "ver"=0) -> ()  [unwired: 7 in, 2 out]
          }
          event "Use": Value Change {
            n670 = event-data() -> ("NewVal"=w824:bool)  [unwired: 1 in, 5 out]
            n671 = local read "Laser"() -> (w822:i16)
            n672 = Increment(x=w822) -> (x+1=w821:i16)
            n673 = Boolean To (0,1)(Boolean=w824) -> (0, 1=w823:i16)
            n674 = dll-call lib="wlmData.dll" fn="SetSwitcherSignalStates"("channel"=w821, "use"=w823) -> ()  [unwired: 6 in, 2 out]
          }
          event "Auto": Value Change {
            n675 = event-data() -> ("NewVal"=w828:bool)  [unwired: 1 in, 5 out]
            n676 = local read "Laser"() -> (w826:i16)
            n677 = Increment(x=w826) -> (x+1=w825:i16)
            n678 = Boolean To (0,1)(Boolean=w828) -> (0, 1=w827:i16)
            n679 = dll-call lib="wlmData.dll" fn="SetExposureModeNum"("num"=w825, "Enable"=w827) -> ()  [unwired: 6 in, 2 out]
          }
          event "Expo.[ms]": Value Change {
            n680 = event-data() -> ("NewVal"=w829:i32[])  [unwired: 1 in, 5 out]
            n681 = local read "Laser"() -> (w831:i16)
            n682 = Increment(x=w831) -> (x+1=w830:i16)
            n683 = call "Expow.vi"("Expo1[ms]"=w829, "Numeric"=w830) -> ()
          }
          event "stop": Value Change {
            n684 = event-data() -> ("NewVal"=w834:bool)  [unwired: 1 in, 5 out]
            n685 = flat-sequence {
              tunnel: w834 -> [w835]
              tunnel: [w835] -> w833
              tunnel: w833 -> [w858]
              tunnel: [w858] -> w832
              frame #0 {
                n686 = local read "Boolean"() -> (w836:bool)
                n687 = case shown="False" w836 {
                  frame False {
                    n688 = dll-call lib="wlmData.dll" fn="ControlWLM"("action"=1, "app"=0, "ver"=0) -> ()  [unwired: 7 in, 2 out]
                    n689 = local read "Boolean 2"() -> (w840:bool)
                    n690 = case shown="False" w840 {
                      frame False {
                        w843 = u16 0 items=["GetText", "Click"] ("Message")
                        n691 = call "FindButton.vi"() -> ("Handle"=w841:u64)
                        n692 = call "startstop.vi"("Message"=w843, "Handle"=w841) -> ("Output"=w845:variant)  [unwired: 1 in]
                        n693 = Variant To Data(type="", Variant=w845) -> (data=w842:string)  [unwired: 1 in, 1 out]
                        n694 = case shown="\"&Stop\"" w842 {
                          tunnel: w841 -> [w846 _]
                          frame Default {
                            w847 = u16 1 items=["GetText", "Click"] ("Message")
                            n695 = call "startstop.vi"("Message"=w847, "Handle"=w846) -> ()  [unwired: 1 in, 1 out]
                          }
                          frame "&Stop" {
                          }
                        }
                      }
                      frame True {
                        w850 = u16 0 items=["GetText", "Click"] ("Message")
                        n696 = call "FindButton.vi"() -> ("Handle"=w848:u64)
                        n697 = call "startstop.vi"("Message"=w850, "Handle"=w848) -> ("Output"=w852:variant)  [unwired: 1 in]
                        n698 = Variant To Data(type="", Variant=w852) -> (data=w849:string)  [unwired: 1 in, 1 out]
                        n699 = case shown="\"&Start\"" w849 {
                          tunnel: w848 -> [w853 _]
                          frame Default {
                            w854 = u16 1 items=["GetText", "Click"] ("Message")
                            n700 = call "startstop.vi"("Message"=w854, "Handle"=w853) -> ()  [unwired: 1 in, 1 out]
                          }
                          frame "&Start" {
                          }
                        }
                      }
                    }
                  }
                  frame True {
                    n701 = dll-call lib="wlmData.dll" fn="ControlWLM"("action"=3, "app"=0, "ver"=0) -> ()  [unwired: 7 in, 2 out]
                  }
                }
              }
              frame #1 {
              }
            }
          }
        }
      }
    }
    frame #3 {
      n702 = VISA Close(VISA resource name=w1105) -> (error out=w1096:errorcluster)  [unwired: 1 in]
      n703 = VISA Close(VISA resource name=w1106) -> (error out=w1095:errorcluster)  [unwired: 1 in]
      n704 = VISA Close(VISA resource name=w1103) -> (error out=w1094:errorcluster)  [unwired: 1 in]
      n705 = VISA Close(VISA resource name=w1104) -> (error out=w1093:errorcluster)  [unwired: 1 in]
      n706 = TCP Close Connection(connection ID=w1110) -> (error out=w1092:errorcluster)  [unwired: 2 in, 1 out]
      n707 = TCP Close Connection(connection ID=w1107) -> (error out=w1089:errorcluster)  [unwired: 2 in, 1 out]
      n708 = TCP Close Connection(connection ID=w1109) -> (error out=w1091:errorcluster)  [unwired: 2 in, 1 out]
      n709 = TCP Close Connection(connection ID=w1108) -> (error out=w1090:errorcluster)  [unwired: 2 in, 1 out]
      n710 = local read "Oscilloscope Error"() -> (w1088:errorcluster)
      n711 = call <vilib>:"Clear Errors.vi"("error in (no error)"=w1096) -> ()  [unwired: 5 in, 2 out]
      n712 = call <vilib>:"Clear Errors.vi"("error in (no error)"=w1092) -> ()  [unwired: 5 in, 2 out]
      n713 = call <vilib>:"Clear Errors.vi"("error in (no error)"=w1095) -> ()  [unwired: 5 in, 2 out]
      n714 = call <vilib>:"Clear Errors.vi"("error in (no error)"=w1094) -> ()  [unwired: 5 in, 2 out]
      n715 = call <vilib>:"Clear Errors.vi"("error in (no error)"=w1089) -> ()  [unwired: 5 in, 2 out]
      n716 = VISA Write(VISA resource name=w1101, write buffer="LOCAL\n") -> (VISA resource name out=w1100:refnum<visa-resource-name>, error out=w1098:errorcluster)  [unwired: 1 in, 1 out]
      n717 = call <vilib>:"Clear Errors.vi"("error in (no error)"=w1093) -> ()  [unwired: 5 in, 2 out]
      n718 = call <vilib>:"Clear Errors.vi"("error in (no error)"=w1091) -> ()  [unwired: 5 in, 2 out]
      n719 = call <vilib>:"Clear Errors.vi"("error in (no error)"=w1090) -> ()  [unwired: 5 in, 2 out]
      n720 = VISA Close(VISA resource name=w1100, error in (no error)=w1098) -> (error out=w1097:errorcluster)
      n721 = call <vilib>:"Clear Errors.vi"("error in (no error)"=w1097) -> ()  [unwired: 5 in, 2 out]
      n722 = case shown="No Error" w1088 {
        tunnel: w1099 -> [_ w1112]
        frame No Error {
        }
        frame Error {
          n723 = VISA Close(VISA resource name=w1112) -> (error out=w1111:errorcluster)  [unwired: 1 in]
          n724 = call <vilib>:"Clear Errors.vi"("error in (no error)"=w1111) -> ()  [unwired: 5 in, 2 out]
        }
      }
    }
  }
